vi "PI Open Interface of one system.vi"(0 "System number":i32=1 min=1 step=1, 2 "Interface clear":string="XXX\n", 3 "Interface configuration":T10={"RS232 Portnumber"=0, "Timeout"=5000, "RS232 Baud rate"=57600, "Interface"=0, "GPIB Bus"=0, "GPIB Address"=4, "GPIB Mode"=0} {"Interface" items=["RS232", "GPIB", "DLL", "TCP-IP", "USB", "Analog"]; "RS232 Portnumber" items=["COM1", "COM2", "COM3", "COM4", "COM5", "COM6", "COM7", "COM8", "COM9", "COM10", "COM11", "COM12", "COM13", "COM14", "COM15", "COM16", "COM17", "COM18", "COM19", "COM20", "COM21", "COM22", "COM23", "COM24", "COM25", "COM26", "COM27", "COM28", "COM29", "COM30"]}, 4 "String to Send":string="*idn?", 5 "error in":errorcluster, 6 "DLL Interface\nConfiguration":T8={"DLL for Device"=0, "DLL Interface"=2, "Parameter"="1"} {"DLL Interface" items=["RS232", "GPIB", "Board", "TCP-IP", "USB", "RS232_DC", "USB_DC", "TCPIP_DC"]; "DLL for Device" items=["C-843", "C-844", "E-710", "C-843.PM", "C-865", "E-761", "Mercury", "E-755", "E-753", "C-866", "E-712", "E-725", "E-861", "C-867", "E-517", "E-816", "E-709", "PI_GCS2_DLL", "HydraPollux"]}, 7 "Bit settings and parity":T4={"data bits"=8, "stop bits"=enum."1 bit", "parity"=enum."no parity"} {"data bits" min=5 max=8 step=1}, 8 "TCP/IP\nConfiguration":T3={"Host address/name"="localhost", "Port"=3000, "Board"=0}, 9 "Flow control":T5={"input XON/XOFF"=FALSE, "input HW Handshake"=FALSE, "input alt HW HShk"=FALSE, "output XON/XOFF"=FALSE, "output HW Handshake"=FALSE, "output alt HW HShk"=FALSE, "XOFF byte "=19, "XON byte"=17, "parity error byte"=0} {"parity error byte" format="%.0x"; "XON byte" format="%.0x"; "XOFF byte" format="%.0x"}, 10 "Termination character":T2, 11 "Syntax":T1, 12 "Register DC":bool) -> (14 "String read":string, 19 "error out":errorcluster)   [LabVIEW 2020]
doc: "Establishes communication with one connected system. This VI is called automatically by PI_GCS2_Configuration_Setup.vi and must be completed successfully before any other VI can use the interface. The interface and error status of the chosen system are cleared by this VI, which sends XXX (no command), *IDN? and ERR?. \n\nC-413: Interface = RS232, DLL, or TCP/IP (TCP/IP support available depending on controller version! If unsure whether your controller supports TCP/IP communication, please refer to the controller user manual). RS232: Input and output HW handshake must be TRUE. DLL: DLL for Device = PI_GCS2_DLL, DLL Interface = USB, Parameter = Serial no. of system to connect to. Syntax: GCS 2.0; Term char = LF.\n\nC-702: Interface = RS232 or TCP/IP, RS232: Input and output HW handshake must be TRUE, Syntax: GCS 1.0; Term char = LF.\n\nC-843: Interface = DLL, DLL for Device = C-843, DLL Interface = Board, Parameter = Board number (1 for first C-843 board), Syntax: GCS 1.0; Term char = LF.\n\nC-843.PM: Interface = DLL, DLL for Device = C-843.PM, DLL Interface = Board, Parameter = Board number (1 for first C-843 board) , Syntax: GCS 1.0; Term char = LF.\n\nC-844: Interface = DLL, DLL for Device = C-844, DLL Interface = RS232 or GPIB, Parameter = empty string, RS232 baud rate = 9600\n\nC-865: Interface = DLL, DLL for Device = C-865, DLL Interface = RS232, Parameter = empty string, RS232 baud rate = set as appropriate, Syntax: GCS 1.0; Term char = LF.\n\nC-866: Interface = DLL, DLL for Device = C-866, DLL Interface = RS232 or USB, RS232: Parameter = empty string, RS232 baud rate = set as appropriate, USB: Parameter = Serial no. of system to connect to, \nSyntax: GCS 1.0; Term char = LF.\n\nC-867: Single Device: Interface = RS232, TCP/IP or DLL, RS232: Input and output HW handshake must be FALSE. DLL (USB): DLL for Device = C-867, DLL Interface = USB, Parameter = Serial no. of system to connect to.\nDaisyChain: Interface = DLL, DLL for Device = C-867, DLL Interface = RS232_DC, Parameter = Number of device in chain, Register DC: FALSE. Syntax: GCS 2.0; Term char = LF.\n\nC-877: Interface = RS232 or DLL, RS232: Input and output HW handshake must be FALSE. DLL (USB): DLL for Device = PI_GCS2_DLL, DLL Interface = USB, Parameter = Serial no. of system to connect to. Syntax: GCS 2.0; Term char = LF.\n\nC-880: Interface = RS232 or GPIB, RS232: Input and output HW handshake must be TRUE, Syntax: GCS 1.0; Term char = LF.\n\nC-848: Interface = RS232 or GPIB, RS232: Input and output HW handshake must be TRUE, Syntax: GCS 1.0; Term char = LF.\n\nC-880K005: Interface = RS232, Input and output HW handshake must be FALSE, Syntax: GCS 1.0; Term char = LF.\n\nC-884: Interface = RS232, TCP/IP or DLL, RS232: Input and output HW handshake must be TRUE. DLL (USB): DLL for Device = PI_GCS2_DLL, DLL Interface = USB, Parameter = Serial no. of system to connect to. Syntax: GCS 2.0; Term char = LF.\n\nC-885: Interface = TCP/IP or DLL. DLL (USB): DLL for Device = PI_GCS2_DLL, DLL Interface = USB, Parameter = Serial no. of system to connect to. Syntax: GCS 2.0; Term char = LF.DaisyChain: Interface = DLL, DLL for Device = PI_GCS2_DLL, DLL Interface = TCPIP_DC or USB_DC, Parameter = Number of device in chain, Register DC: FALSE. Syntax: GCS 2.0; Term char = LF.\n\nC-886: Interface = TCP/IP or DLL. DLL (USB): DLL for Device = PI_GCS2_DLL, DLL Interface = USB, Parameter = Serial no. of system to connect to. Syntax: GCS 2.0; Term char = LF.\n\nC-891: Interface = RS232, TCP/IP or DLL. TCP/IP support available depending on controller version! If unsure whether your controller supports TCP/IP communication, please refer to your user manual.RS232: Input and output HW handshake must be FALSE. DLL: DLL for Device = C-891, DLL Interface = USB, Parameter = Serial no. of system to connect to. Syntax: GCS 2.0; Term char = LF.\n\nE-135: Interface = RS232, DLL, or TCP/IP. RS232: Input and output HW handshake must be TRUE. DLL: DLL for Device = PI_GCS2_DLL, DLL Interface = USB, Parameter = Serial no. of system to connect to. Syntax: GCS 2.0; Term char = LF.\n\nE-516: Interface = RS232 or GPIB, RS232: Input and output HW handshake must be TRUE, Syntax: GCS 1.0; Term char = LF.\n\nE-517: Interface = RS232, GPIB, TCP/IP or DLL, RS232: Input and output HW handshake must be TRUE, DLL (USB): DLL for Device = E-517, DLL Interface = USB, Parameter = Serial no. of system to connect to. Syntax: GCS 2.0; Term char = LF.\n\nE-518: Interface = RS232, TCP/IP or DLL, RS232: Input and output HW handshake must be TRUE, DLL (USB): DLL for Device = PI_GCS2_DLL, DLL Interface = SB, Parameter = Serial no. of system to connect to. Syntax: GCS 2.0; Term char = LF.\n\nE-709: Interface = RS232 or USB, RS232: Input and output HW handshake must be TRUE, DLL: DLL for Device = E-709, DLL Interface = USB, Parameter = Serial no. of system to connect to. \nSyntax: GCS 2.0; Term char = LF.\n\nE-710: Interface = DLL, DLL for Device = E-710, DLL Interface = RS232 or GPIB, Parameter = empty string, Syntax: GCS 1.0; Term char = LF.\n\nE-712: Interface = RS232, TCP/IP or DLL, RS232: Input and output HW handshake must be TRUE. DLL: DLL for Device = E-712, DLL Interface = USB, Parameter = Serial no. of system to connect to. Syntax: GCS 2.0; Term char = LF.\n\nE-725: Interface = RS232, TCP/IP or DLL, RS232: Input and output HW handshake must be TRUE. DLL: DLL for Device = E-725, DLL Interface = USB, Parameter = Serial no. of system to connect to. Syntax: GCS 2.0; Term char = LF.\n\nE-727: Interface = RS232, TCP/IP or DLL, RS232: Input and output HW handshake must be TRUE. DLL: DLL for Device = PI_GCS2_DLL, DLL Interface = USB, arameter = Serial no. of system to connect to. Syntax: GCS 2.0; Term char = LF.\n\nE-753: Interface = RS232 or TCP/IP, RS232: Input and output HW handshake must be TRUE, Syntax: GCS 2.0; Term char = LF.\n\nE-754: Interface = RS232, TCP/IP or DLL, RS232: Input and output HW handshake must be TRUE. DLL: DLL for Device = E-754, DLL Interface = USB, Parameter = Serial no. of system to connect to. Syntax: GCS 2.0; Term char = LF.\n\nE-755: Single Device: Interface = RS232, Input and output HW handshake must be TRUE.\nDaisyChain: Interface = DLL, DLL for Device = E-755, DLL Interface = RS232_DC, Parameter = Number of device in chain (first device: 1), Register DC: FALSE.\nSyntax: GCS 2.0; Term char = LF.\n\nE-761: Interface = DLL, DLL for Device = E-761, DLL Interface = Board, Parameter = Board number (1 for first E-761 board), Syntax: GCS 1.0; Term char = LF.\n\nE-816: Interface = RS232 or DLL, RS232: Input and output HW handshake must be TRUE. DLL (USB): DLL for Device = E-816, DLL Interface = USB, Parameter = Serial no. of system to connect to. Syntax: GCS 1.0; Term char = LF. \n\nE-861: Single Device: Interface = RS232 or DLL, RS232: Input and output HW handshake must be FALSE. DLL (USB): DLL for Device = E-861, DLL Interface = USB, Parameter = Serial no. of system to connect to.\nDaisyChain: Interface = DLL, DLL for Device = E-861, DLL Interface = RS232_DC or USB_DC, Parameter = Number of device in chain, Register DC: FALSE. Syntax: GCS 2.0; Term char = LF.\n\nE-870: Interface = DLL, DLL (USB): DLL for Device = PI_GCS2_DLL, DLL Interface = USB, Parameter = Serial no. of system to connect to. Syntax: GCS 2.0; Term char = LF. \n\nE-871: Single Device: Interface = RS232 or DLL, RS232: Input and output HW handshake must be FALSE. DLL (USB): DLL for Device = PI_GCS2_DLL, DLL Interface = USB, Parameter = Serial no. of system to connect to.\nDaisyChain: Interface = DLL, DLL for Device = PI_GCS2_DLL, DLL Interface = RS232_DC or USB_DC, Parameter = Number of device in chain, Register DC: FALSE. Syntax: GCS 2.0; Term char = LF.\n\nE-872: Interface = RS232, TCP/IP or DLL, RS232: Input and output HW handshake must be FALSE. DLL (USB): DLL for Device = PI_GCS2_DLL, DLL Interface = USB, Parameter = Serial no. of system to connect to. Syntax: GCS 2.0; Term char = LF.\n\nE-873: Interface = RS232, TCP/IP or DLL, RS232: Input and output HW handshake must be FALSE. DLL (USB): DLL for Device = PI_GCS2_DLL, DLL Interface = USB, Parameter = Serial no. of system to connect to. Syntax: GCS 2.0; Term char = LF.\n\nE-874: Interface = RS232, TCP/IP or DLL, RS232: Input and output HW handshake must be FALSE. DLL (USB): DLL for Device = PI_GCS2_DLL, DLL Interface = USB, Parameter = Serial no. of system to connect to. Syntax: GCS 2.0; Term char = LF.\n\nF-206: F-206 (GCS 1.0): Interface = RS232, GPIB or TCP/IP, The error status will not be cleared by this VI. The first ERR? query will report a hidden error with error code 1, which will be cleared during system initialization (INI). RS232: Input and output handshake settings must be FALSE, Syntax: GCS 1.0; Term char = LF.\n\nC-887 + H-206 (GCS 2.0): Interface = RS232 or TCP/IP, RS232: Input and output handshake settings must be FALSE, Syntax: GCS 2.0; Term char = LF.\n\nHydra: Interface = DLL, DLL (TCP/IP and RS-232): DLL for Device = PI_HydraPollux_GCS2_DLL, DLL Interface = RS232 or TCP/IP, Syntax: GCS 2.0; Term char = LF. \n\nM-8X0: M-810/11/24/40/50 (GCS 1.0): Interface = RS232, GPIB or TCP/IP, RS232: Input and output handshake settings must be FALSE, Syntax: GCS 1.0; Term char = LF.\n\nC-887 + H-810/11/24/40/50 (GCS 2.0): Interface = RS232 or TCP/IP, RS232: Input and output handshake settings must be FALSE, Syntax: GCS 2.0; Term char = LF.\n\nMercury: Interface = DLL, DLL for Device = Mercury, DLL Interface = RS232 (even if using USB), Parameter = empty string, RS232 baud rate = same as controller hardware setting (even if using USB), Syntax: GCS 1.0; Term char = LF.\n\nMercury_GCS: Single Device: Interface = RS232 or DLL, RS232: Input and output HW handshake must be FALSE. DLL (USB): DLL for Device = PI_GCS2_DLL, DLL Interface = USB, Parameter = Serial no. of system to connect to.\nDaisyChain: Interface = DLL, DLL for Device = PI_GCS2_DLL, DLL Interface = RS232_DC or USB_DC, Parameter = Number of device in chain, Register DC: FALSE. Syntax: GCS 2.0; Term char = LF.\n\nPollux: Interface = DLL, DLL (RS-232): DLL for Device = PI_HydraPollux_GCS2_DLL, DLL Interface = RS232, Baudrate must be 19200. Syntax: GCS 2.0; Term char = LF."
uses:
  Available interfaces.ctl
  Available DLLs.ctl
  Available DLL interfaces.ctl
  Termination character.ctl
  Syntax.ctl
  Global1.vi
  <vilib>/Instr/_visa.llb/VISA Configure Serial Port (Instr).vi
panel:
  out "DLL device ID":i32 caption="error code"
  # "Establishes communication with one connected system. This VI is called automatically by \"XXXX_\nConfiguration_Setup.vi\" (with XXXX being the PI product number of your system) and must be \ncompleted successfully before any other VI can use the interface. The interface and error status \nof the chosen system are cleared by this VI, which sends XXX (no command), *IDN? and ERR?. \nOther system entries are not touched."
  # "Other parameters:"
  # "TCP/IP:"
  # "DLL:"
  # "General:"
  # "RS232:"
  # "GPIB:"
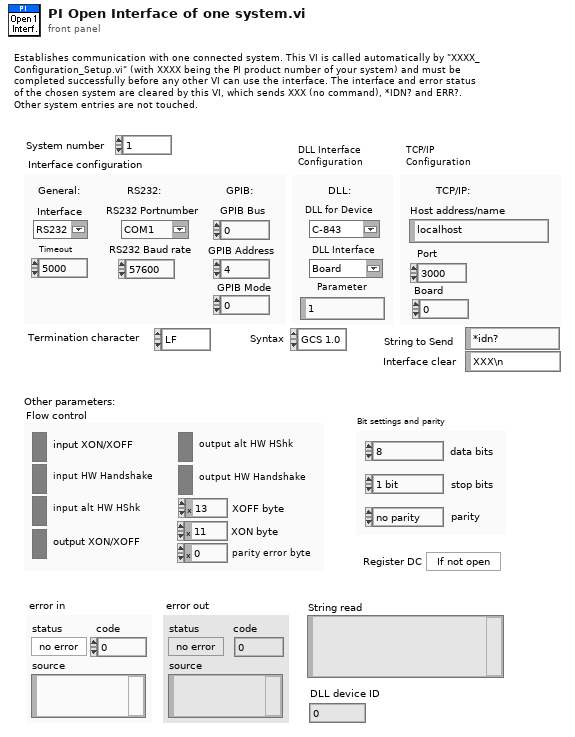
[diagram p1: front panel]
types:
  T1 = typedef "Syntax.ctl" = enum16{"GCS 1.0", "GCS 2.0", "GCS 3.0"}
  T2 = typedef "Termination character.ctl" = enum16{"LF", "CR", "LFCR", "CRLF"}
  T3 = cluster{"Host address/name":string, "Port":i32, "Board":i32}
  T4 = cluster{"data bits":u16, "stop bits":enum16{"1 bit", "1.5 bits", "2 bits"}, "parity":enum16{"no parity", "odd parity", "even parity", "mark parity", "space parity"}}
  T5 = cluster{"input XON/XOFF":bool, "input HW Handshake":bool, "input alt HW HShk":bool, "output XON/XOFF":bool, "output HW Handshake":bool, "output alt HW HShk":bool, "XOFF byte ":u8, "XON byte":u8, "parity error byte":u16}
  T6 = typedef "Available DLLs.ctl" = u16
  T7 = typedef "Available DLL interfaces.ctl" = u16
  T8 = cluster{"DLL for Device":T6, "DLL Interface":T7, "Parameter":string}
  T9 = typedef "Available interfaces.ctl" = u16
  T10 = cluster{"RS232 Portnumber":i32, "Timeout":i32, "RS232 Baud rate":u32, "Interface":T9, "GPIB Bus":i32, "GPIB Address":i32, "GPIB Mode":i32}
  T11 = enum16{"C844_IsDLLAvailable", "C844_ConnectRS232", "C844_ConnectNIgpib", "C844_IsConnected", "C844_CloseConnection", "C844_GcsCommandset", "C844_GetError", "C844_GcsGetAnswerSize", "C844_GcsGetAnswer", "C843_IsDLLAvailable", "C843_Connect", "C843_IsConnected", "C843_CloseConnection", "C843_GcsCommandset", "C843_GetError", "C843_GcsGetAnswerSize", "C843_GcsGetAnswer", "E710_IsDLLAvailable", "E710_ConnectRS232", "E710_ConnectNIgpib", "E710_IsConnected", "E710_CloseConnection", "E710_GcsCommandset", "E710_GetError", "E710_GcsGetAnswerSize", "E710_GcsGetAnswer", "C843_PM_IsDLLAvailable", "C843_PM_Connect", "C843_PM_IsConnected", "C843_PM_CloseConnection", "C843_PM_GcsCommandset", "C843_PM_GetError", "C843_PM_GcsGetAnswerSize", "C843_PM_GcsGetAnswer", "C843_PM_GetCurrentBoardID", "C843_GetCurrentBoardID", "C865_IsDLLAvailable", "C865_ConnectRS232", "C865_IsConnected", "C865_CloseConnection", "C865_GcsCommandset", "C865_GetError", "C865_GcsGetAnswerSize", "C865_GcsGetAnswer", "C865_GetCurrentInterfaceID", "E761_ConnectPciBoard", "DefineSystem", "CloseConnection", "IsConnected", "ConnectRS232", "ConnectNIgpib", "ConnectPciBoard", "ConnectTCPIP", "GetError", "GcsCommandset", "GCSGetAnswerSize", "GcsGetAnswer"}
  T12 = enum16{"C844_IsDLLAvailable", "C844_ConnectRS232", "C844_ConnectNIgpib", "C844_IsConnected", "C844_CloseConnection", "C844_GcsCommandset", "C844_GetError", "C844_GcsGetAnswerSize", "C844_GcsGetAnswer", "C843_IsDLLAvailable", "C843_Connect", "C843_IsConnected", "C843_CloseConnection", "C843_GcsCommandset", "C843_GetError", "C843_GcsGetAnswerSize", "C843_GcsGetAnswer", "E710_IsDLLAvailable", "E710_ConnectRS232", "E710_ConnectNIgpib", "E710_IsConnected", "E710_CloseConnection", "E710_GcsCommandset", "E710_GetError", "E710_GcsGetAnswerSize", "E710_GcsGetAnswer", "C843_PM_IsDLLAvailable", "C843_PM_Connect", "C843_PM_IsConnected", "C843_PM_CloseConnection", "C843_PM_GcsCommandset", "C843_PM_GetError", "C843_PM_GcsGetAnswerSize", "C843_PM_GcsGetAnswer", "C843_PM_GetCurrentBoardID", "C843_GetCurrentBoardID", "C865_IsDLLAvailable", "C865_ConnectRS232", "C865_IsConnected", "C865_CloseConnection", "C865_GcsCommandset", "C865_GetError", "C865_GcsGetAnswerSize", "C865_GcsGetAnswer", "C865_GetCurrentInterfaceID", "E761_ConnectPciBoard", "DefineSystem", "CloseConnection", "IsConnected", "ConnectRS232", "ConnectNIgpib", "ConnectPciBoard", "ConnectTCPIP", "GetError", "GcsCommandset", "GCSGetAnswerSize", "GcsGetAnswer", "CloseDaisyChain", "OpenRS232DaisyChain", "ConnectDaisyChainDevice", "ConnectUSB", "ListUSB"}
  T13 = enum16{"C844_IsDLLAvailable", "C844_ConnectRS232", "C844_ConnectNIgpib", "C844_IsConnected", "C844_CloseConnection", "C844_GcsCommandset", "C844_GetError", "C844_GcsGetAnswerSize", "C844_GcsGetAnswer", "C843_IsDLLAvailable", "C843_Connect", "C843_IsConnected", "C843_CloseConnection", "C843_GcsCommandset", "C843_GetError", "C843_GcsGetAnswerSize", "C843_GcsGetAnswer", "E710_IsDLLAvailable", "E710_ConnectRS232", "E710_ConnectNIgpib", "E710_IsConnected", "E710_CloseConnection", "E710_GcsCommandset", "E710_GetError", "E710_GcsGetAnswerSize", "E710_GcsGetAnswer", "C843_PM_IsDLLAvailable", "C843_PM_Connect", "C843_PM_IsConnected", "C843_PM_CloseConnection", "C843_PM_GcsCommandset", "C843_PM_GetError", "C843_PM_GcsGetAnswerSize", "C843_PM_GcsGetAnswer", "C843_PM_GetCurrentBoardID", "C843_GetCurrentBoardID", "C865_IsDLLAvailable", "C865_ConnectRS232", "C865_IsConnected", "C865_CloseConnection", "C865_GcsCommandset", "C865_GetError", "C865_GcsGetAnswerSize", "C865_GcsGetAnswer", "C865_GetCurrentInterfaceID", "E761_ConnectPciBoard", "DefineSystem", "CloseConnection", "IsConnected", "ConnectRS232", "ConnectNIgpib", "ConnectPciBoard", "ConnectTCPIP", "GetError", "GcsCommandset", "GCSGetAnswerSize", "GcsGetAnswer", "CloseDaisyChain", "OpenRS232DaisyChain", "ConnectDaisyChainDevice"}
  T14 = enum16{"C844_IsDLLAvailable", "C844_ConnectRS232", "C844_ConnectNIgpib", "C844_IsConnected", "C844_CloseConnection", "C844_GcsCommandset", "C844_GetError", "C844_GcsGetAnswerSize", "C844_GcsGetAnswer", "C843_IsDLLAvailable", "C843_Connect", "C843_IsConnected", "C843_CloseConnection", "C843_GcsCommandset", "C843_GetError", "C843_GcsGetAnswerSize", "C843_GcsGetAnswer", "E710_IsDLLAvailable", "E710_ConnectRS232", "E710_ConnectNIgpib", "E710_IsConnected", "E710_CloseConnection", "E710_GcsCommandset", "E710_GetError", "E710_GcsGetAnswerSize", "E710_GcsGetAnswer", "C843_PM_IsDLLAvailable", "C843_PM_Connect", "C843_PM_IsConnected", "C843_PM_CloseConnection", "C843_PM_GcsCommandset", "C843_PM_GetError", "C843_PM_GcsGetAnswerSize", "C843_PM_GcsGetAnswer", "C843_PM_GetCurrentBoardID", "C843_GetCurrentBoardID", "C865_IsDLLAvailable", "C865_ConnectRS232", "C865_IsConnected", "C865_CloseConnection", "C865_GcsCommandset", "C865_GetError", "C865_GcsGetAnswerSize", "C865_GcsGetAnswer", "C865_GetCurrentInterfaceID", "E761_ConnectPciBoard", "DefineSystem", "CloseConnection", "IsConnected", "ConnectRS232", "ConnectNIgpib", "ConnectPciBoard", "ConnectTCPIP", "GetError", "GcsCommandset", "GCSGetAnswerSize", "GcsGetAnswer", "CloseDaisyChain", "OpenRS232DaisyChain", "ConnectDaisyChainDevice", "ConnectUSB", "ListUSB", "OpenUSBDaisyChain"}
  T15 = enum16{"C844_IsDLLAvailable", "C844_ConnectRS232", "C844_ConnectNIgpib", "C844_IsConnected", "C844_CloseConnection", "C844_GcsCommandset", "C844_GetError", "C844_GcsGetAnswerSize", "C844_GcsGetAnswer", "C843_IsDLLAvailable", "C843_Connect", "C843_IsConnected", "C843_CloseConnection", "C843_GcsCommandset", "C843_GetError", "C843_GcsGetAnswerSize", "C843_GcsGetAnswer", "E710_IsDLLAvailable", "E710_ConnectRS232", "E710_ConnectNIgpib", "E710_IsConnected", "E710_CloseConnection", "E710_GcsCommandset", "E710_GetError", "E710_GcsGetAnswerSize", "E710_GcsGetAnswer", "C843_PM_IsDLLAvailable", "C843_PM_Connect", "C843_PM_IsConnected", "C843_PM_CloseConnection", "C843_PM_GcsCommandset", "C843_PM_GetError", "C843_PM_GcsGetAnswerSize", "C843_PM_GcsGetAnswer", "C843_PM_GetCurrentBoardID", "C843_GetCurrentBoardID", "C865_IsDLLAvailable", "C865_ConnectRS232", "C865_IsConnected", "C865_CloseConnection", "C865_GcsCommandset", "C865_GetError", "C865_GcsGetAnswerSize", "C865_GcsGetAnswer", "C865_GetCurrentInterfaceID", "E761_ConnectPciBoard", "DefineSystem", "CloseConnection", "IsConnected", "ConnectRS232", "ConnectNIgpib", "ConnectPciBoard", "ConnectTCPIP", "GetError", "GcsCommandset", "GCSGetAnswerSize", "GcsGetAnswer", "CloseDaisyChain", "OpenRS232DaisyChain", "ConnectDaisyChainDevice", "ConnectUSB", "ListUSB", "OpenUSBDaisyChain", "OpenTCPIPDaisyChain"}
  T16 = enum16{"C844_IsDLLAvailable", "C844_ConnectRS232", "C844_ConnectNIgpib", "C844_IsConnected", "C844_CloseConnection", "C844_GcsCommandset", "C844_GetError", "C844_GcsGetAnswerSize", "C844_GcsGetAnswer", "C843_IsDLLAvailable", "C843_Connect", "C843_IsConnected", "C843_CloseConnection", "C843_GcsCommandset", "C843_GetError", "C843_GcsGetAnswerSize", "C843_GcsGetAnswer"}
  T17 = enum16{"C844_IsDLLAvailable", "C844_ConnectRS232", "C844_ConnectNIgpib", "C844_IsConnected", "C844_CloseConnection", "C844_GcsCommandset", "C844_GetError", "C844_GcsGetAnswerSize", "C844_GcsGetAnswer"}
  T18 = enum16{"C844_IsDLLAvailable", "C844_ConnectRS232", "C844_ConnectNIgpib", "C844_IsConnected", "C844_CloseConnection", "C844_GcsCommandset", "C844_GetError", "C844_GcsGetAnswerSize", "C844_GcsGetAnswer", "C843_IsDLLAvailable", "C843_Connect", "C843_IsConnected", "C843_CloseConnection", "C843_GcsCommandset", "C843_GetError", "C843_GcsGetAnswerSize", "C843_GcsGetAnswer", "E710_IsDLLAvailable", "E710_ConnectRS232", "E710_ConnectNIgpib", "E710_IsConnected", "E710_CloseConnection", "E710_GcsCommandset", "E710_GetError", "E710_GcsGetAnswerSize", "E710_GcsGetAnswer", "C843_PM_IsDLLAvailable", "C843_PM_Connect", "C843_PM_IsConnected", "C843_PM_CloseConnection", "C843_PM_GcsCommandset", "C843_PM_GetError", "C843_PM_GcsGetAnswerSize", "C843_PM_GcsGetAnswer", "C843_PM_GetCurrentBoardID", "C843_GetCurrentBoardID", "C865_IsDLLAvailable", "C865_ConnectRS232", "C865_IsConnected", "C865_CloseConnection", "C865_GcsCommandset", "C865_GetError", "C865_GcsGetAnswerSize", "C865_GcsGetAnswer", "C865_GetCurrentInterfaceID"}
  T19 = enum16{"C844_IsDLLAvailable", "C844_ConnectRS232", "C844_ConnectNIgpib", "C844_IsConnected", "C844_CloseConnection", "C844_GcsCommandset", "C844_GetError", "C844_GcsGetAnswerSize", "C844_GcsGetAnswer", "C843_IsDLLAvailable", "C843_Connect", "C843_IsConnected", "C843_CloseConnection", "C843_GcsCommandset", "C843_GetError", "C843_GcsGetAnswerSize", "C843_GcsGetAnswer", "E710_IsDLLAvailable", "E710_ConnectRS232", "E710_ConnectNIgpib", "E710_IsConnected", "E710_CloseConnection", "E710_GcsCommandset", "E710_GetError", "E710_GcsGetAnswerSize", "E710_GcsGetAnswer"}
  T20 = enum16{"C844_IsDLLAvailable", "C844_ConnectRS232", "C844_ConnectNIgpib", "C844_IsConnected", "C844_CloseConnection", "C844_GcsCommandset", "C844_GetError", "C844_GcsGetAnswerSize", "C844_GcsGetAnswer", "C843_IsDLLAvailable", "C843_Connect", "C843_IsConnected", "C843_CloseConnection", "C843_GcsCommandset", "C843_GetError", "C843_GcsGetAnswerSize", "C843_GcsGetAnswer", "E710_IsDLLAvailable", "E710_ConnectRS232", "E710_ConnectNIgpib", "E710_IsConnected", "E710_CloseConnection", "E710_GcsCommandset", "E710_GetError", "E710_GcsGetAnswerSize", "E710_GcsGetAnswer", "C843_PM_IsDLLAvailable", "C843_PM_Connect", "C843_PM_IsConnected", "C843_PM_CloseConnection", "C843_PM_GcsCommandset", "C843_PM_GetError", "C843_PM_GcsGetAnswerSize", "C843_PM_GcsGetAnswer"}
  T21 = cluster{"DLL for Device":T6, "DLL Interface":T7, "Parameter":string}[]
  T22 = cluster{"Host address/name":string, "Port":i32, "Board":i32}[]
  T23 = cluster{"RS232 Portnumber":i32, "Timeout":i32, "RS232 Baud rate":u32, "Interface":T9, "GPIB Bus":i32, "GPIB Address":i32, "GPIB Mode":i32}[]
  T24 = cluster{"data bits":u16, "stop bits":enum16{"1 bit", "1.5 bits", "2 bits"}, "parity":enum16{"no parity", "odd parity", "even parity", "mark parity", "space parity"}}[]
  T25 = cluster{"input XON/XOFF":bool, "input HW Handshake":bool, "input alt HW HShk":bool, "output XON/XOFF":bool, "output HW Handshake":bool, "output alt HW HShk":bool, "XOFF byte ":u8, "XON byte":u8, "parity error byte":u16}[]
  T26 = enum16{"no parity", "odd parity", "even parity", "mark parity", "space parity"}
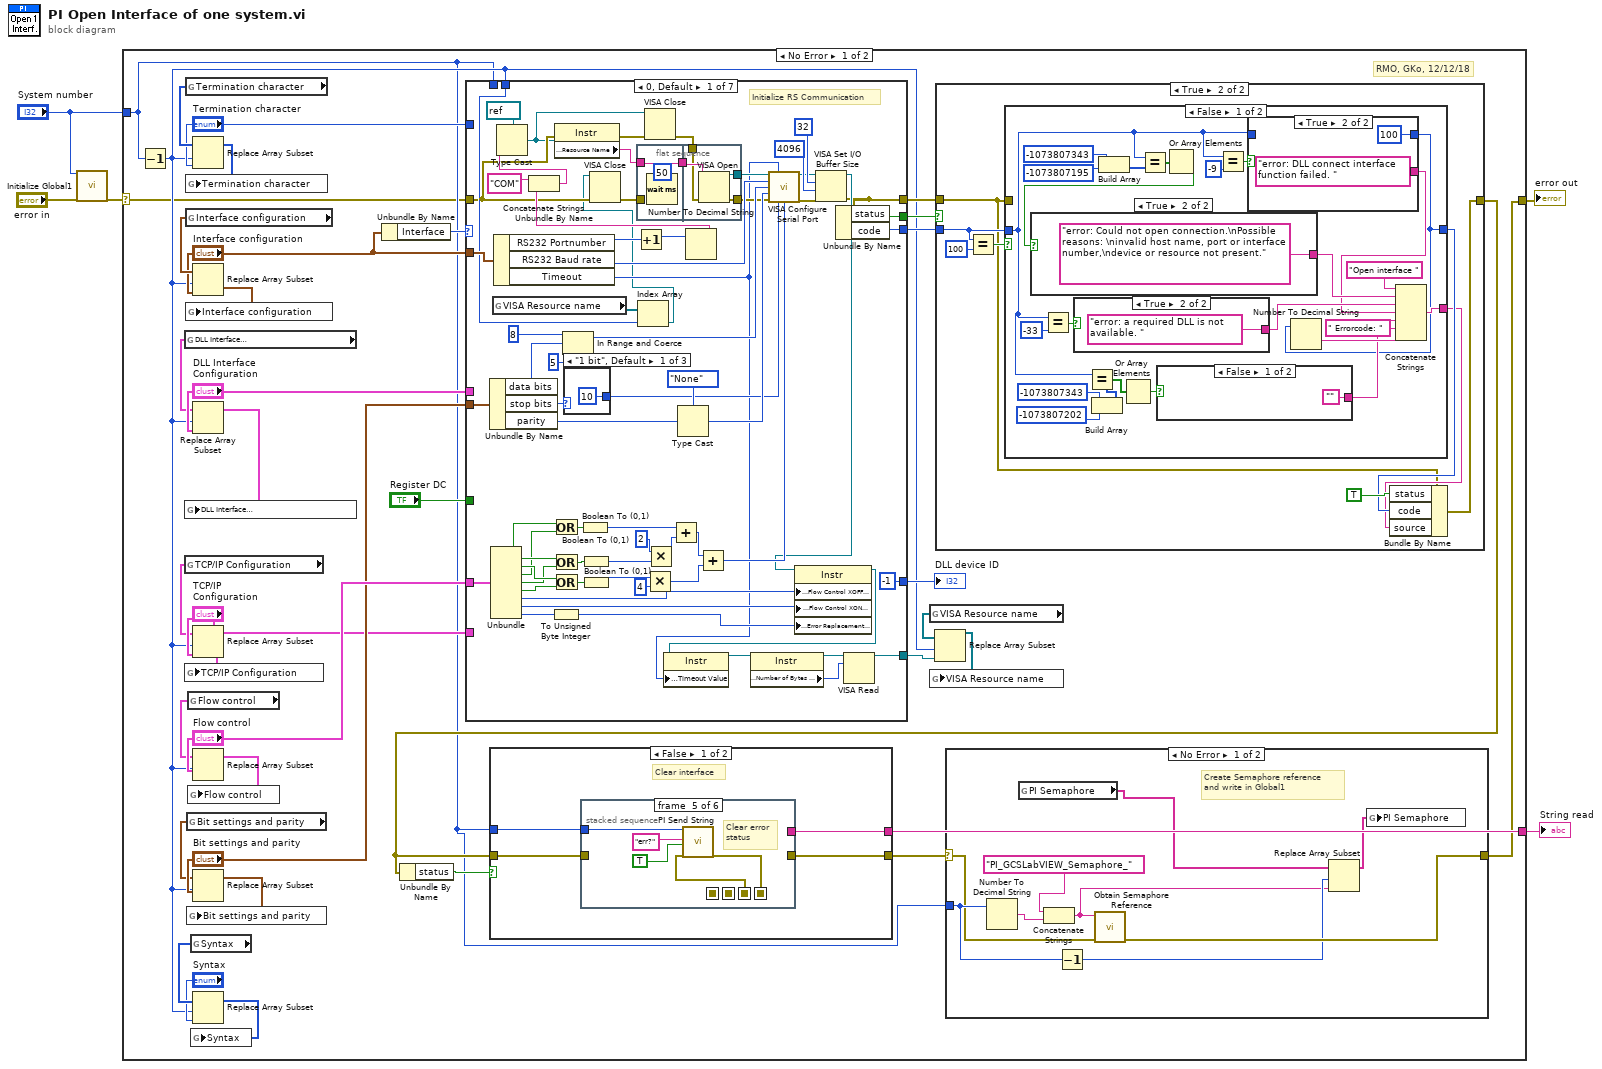
[diagram p0: block diagram]
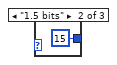
[diagram p3: hidden frame]
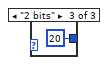
[diagram p4: hidden frame]
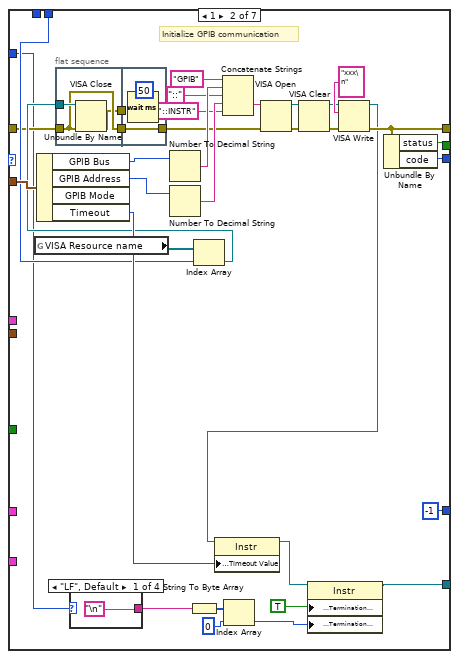
[diagram p5: hidden frame]
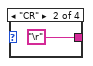
[diagram p6: hidden frame]
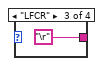
[diagram p7: hidden frame]
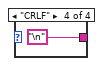
[diagram p8: hidden frame]
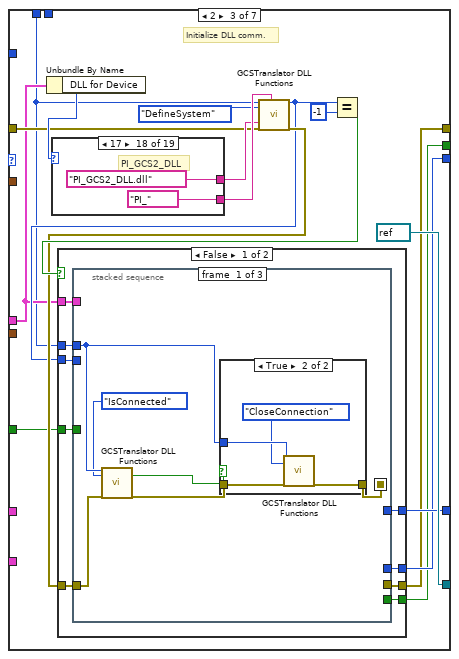
[diagram p9: hidden frame]
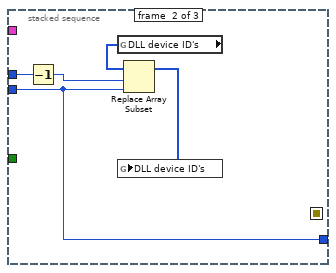
[diagram p11: hidden frame]
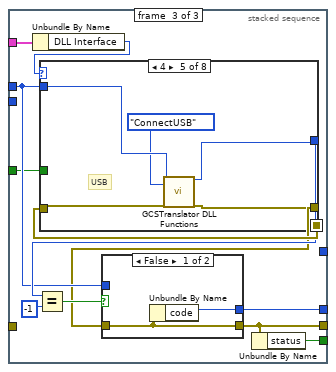
[diagram p12: hidden frame]
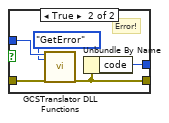
[diagram p13: hidden frame]
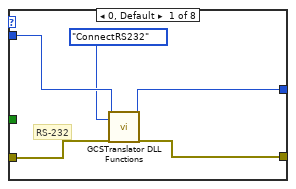
[diagram p14: hidden frame]
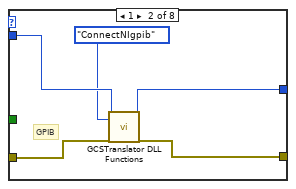
[diagram p15: hidden frame]
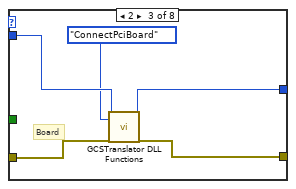
[diagram p16: hidden frame]
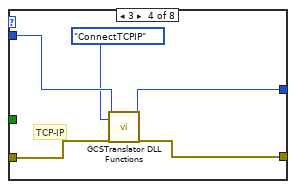
[diagram p17: hidden frame]
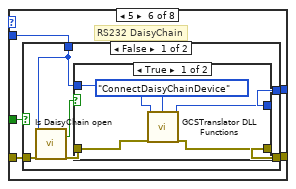
[diagram p18: hidden frame]
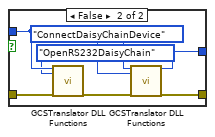
[diagram p19: hidden frame]
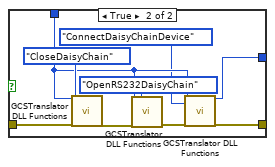
[diagram p20: hidden frame]
diagram:
  n1 = call "Initialize Global1.vi"("System no."="System number", "error in"="error in") -> ("error out"=w1:errorcluster)  [unwired: 17 out]
  n2 = case shown="No Error" w1 {
    selector: w1 -> [w6 w906]
    tunnel: [w8 w906] -> w4
    tunnel: [w29 "" ("String read")] -> w5
    tunnel: "System number" -> [w9 _]
    frame No Error {
      # "RMO, GKo, 12/12/18"
      n3 = Decrement(x=w9) -> (x-1=w11:i32)
      n4 = global read "Global1.vi" "DLL Interface\nConfiguration"() -> (w34:T21)
      n5 = global read "Global1.vi" "TCP/IP Configuration"() -> (w25:T22)
      n6 = global read "Global1.vi" "Termination character"() -> (w18:T2[])
      n7 = global read "Global1.vi" "Interface configuration"() -> (w42:T23)
      n8 = global read "Global1.vi" "Bit settings and parity"() -> (w30:T24)
      n9 = global read "Global1.vi" "Flow control"() -> (w32:T25)
      n10 = global read "Global1.vi" "Syntax"() -> (w15:T1[])
      n11 = Replace Array Subset(array=w18, new element="Termination character", index=w11) -> (w17:T2[])
      n12 = global write "Global1.vi" "Termination character"(w17) -> ()
      n13 = Replace Array Subset(array=w42, new element="Interface configuration", index=w11) -> (w41:T23)
      n14 = global write "Global1.vi" "Interface configuration"(w41) -> ()
      n15 = Replace Array Subset(array=w34, new element="DLL Interface\nConfiguration", index=w11) -> (w38:T21)
      n16 = global write "Global1.vi" "DLL Interface\nConfiguration"(w38) -> ()
      n17 = Replace Array Subset(array=w25, new element="TCP/IP\nConfiguration", index=w11) -> (w21:T22)
      n18 = global write "Global1.vi" "TCP/IP Configuration"(w21) -> ()
      n19 = Replace Array Subset(array=w32, new element="Flow control", index=w11) -> (w33:T25)
      n20 = global write "Global1.vi" "Flow control"(w33) -> ()
      n21 = Replace Array Subset(array=w30, new element="Bit settings and parity", index=w11) -> (w31:T24)
      n22 = global write "Global1.vi" "Bit settings and parity"(w31) -> ()
      n23 = Replace Array Subset(array=w15, new element="Syntax", index=w11) -> (w14:T1[])
      n24 = global write "Global1.vi" "Syntax"(w14) -> ()
      n25 = Unbundle By Name("Interface configuration") -> ("Interface"=w40:T9)
      n26 = case shown="0, Default" w40 {
        tunnel: [w121 w154 w183 w422 0 0 w468] -> w19
        tunnel: "Interface configuration" -> [w119 w165 _ w425 _ _ _]
        tunnel: "DLL Interface\nConfiguration" -> [_ _ w179 _ _ _ w467]
        tunnel: w9 -> [_ _ w176 _ _ _ w461]
        tunnel: [w57 w147 w182 w416 errorcluster {"status"=TRUE, "code"=100, "source"="PI Open Interface of one system.vi:\nUSB interface not supported"} ("error out") w460 w466] -> w28
        tunnel: "Flow control" -> [w87 _ _ _ _ _ _]
        tunnel: "Bit settings and parity" -> [w118 _ _ _ _ _ _]
        tunnel: w6 -> [w65 w139 w187 w404 _ w460 w464]
        tunnel: "TCP/IP\nConfiguration" -> [_ _ _ w434 _ _ _]
        tunnel: [w79 w151 refnum<visa-resource-name> refnum ("duplicate VISA resource name") w423 refnum<visa-resource-name> refnum ("duplicate VISA resource name") refnum<visa-resource-name> refnum ("duplicate VISA resource name") refnum<visa-resource-name> refnum ("duplicate VISA resource name")] -> w22
        tunnel: [-1 -1 w185 -1 0 ("error code") 0 ("error code") w463] -> w20
        tunnel: "Termination character" -> [_ w133 _ w414 _ _ _]
        tunnel: [w72 w141 w178 w406 FALSE ("status") FALSE ("status") w462] -> w12
        tunnel: w11 -> [w71 w140 _ w405 _ _ _]
        tunnel: "Register DC" -> [_ _ w175 _ _ _ _]
        frame 0, Default {
          # "Initialize RS Communication"
          n27 = Unbundle By Name(w118) -> ("data bits"=w111:u16, "stop bits"=w110:enum16{"1 bit", "1.5 bits", "2 bits"}, "parity"=w116:T26)
          n28 = Unbundle(w87) -> ("input XON/XOFF"=w89:bool, "input HW Handshake"=w92:bool, "input alt HW HShk"=w94:bool, "output XON/XOFF"=w90:bool, "output HW Handshake"=w93:bool, "output alt HW HShk"=w95:bool, "XOFF byte"=w106:u8, "XON byte"=w107:u8, "parity error byte"=w88:u16)
          n29 = global read "Global1.vi" "VISA Resource name"() -> (w73:refnum<visa-resource-name>[])
          n30 = Unbundle By Name(w119) -> ("RS232 Portnumber"=w75:i32, "RS232 Baud rate"=w120:u32, "Timeout"=w78:i32)
          n31 = To Unsigned Byte Integer(number=w88) -> (unsigned 8bit integer=w108:u8)
          n32 = Or(x=w89, y=w90) -> (x .or. y?=w91:bool)
          n33 = Or(x=w92, y=w93) -> (x .or. y?=w96:bool)
          n34 = Or(x=w94, y=w95) -> (x .or. y?=w97:bool)
          n35 = In Range and Coerce(upper limit=u16 8, x=w111, lower limit=u16 5) -> (coerced(x)=w112:u16)  [unwired: 1 out]
          n36 = case shown="\"1 bit\", Default" w110 {
            tunnel: [u16 10 u16 15 u16 20] -> w109
            frame "1 bit", Default {
            }
            frame "1.5 bits" {
            }
            frame "2 bits" {
            }
          }
          n37 = Boolean To (0,1)(Boolean=w91) -> (0, 1=w102:i16)
          n38 = Boolean To (0,1)(Boolean=w96) -> (0, 1=w99:i16)
          n39 = Boolean To (0,1)(Boolean=w97) -> (0, 1=w101:i16)
          n40 = Increment(x=w75) -> (x+1=w76:i32)
          n41 = flat-sequence {
            tunnel: w74 -> [_]
            tunnel: w67 -> [w123]
            tunnel: [w123] -> w63
            tunnel: [w127] -> w83
            tunnel: [w126] -> w82
            tunnel: w63 -> [w125]
            tunnel: w54 -> [w124]
            frame #0 {
              n42 = Wait (ms)(milliseconds to wait=u32 50) -> ()  [unwired: 1 out]
            }
            frame #1 {
              n43 = VISA Open(error in (no error)=w124, VISA resource name=w125) -> (VISA resource name=w127:refnum<visa-resource-name>, error out=w126:errorcluster)  [unwired: 3 out]
            }
          }
          n44 = Index Array(array=w73, index=w71) -> (element=w64:refnum<visa-resource-name>)
          n45 = VISA Close(VISA resource name=w64, error in (no error)=w65) -> (error out=w74:errorcluster)
          n46 = Multiply(x=w101, y=u16 4) -> (x*y=w104:u16)
          n47 = Multiply(x=u16 2 ("y"), y=w99) -> (x*y=w103:u16)
          n48 = Add(x=w102, y=w103) -> (x+y=w105:u16)
          n49 = Type Cast(type=enum16{"None", "Odd", "Even", "Mark", "Space"}."None" ("parity (0:none)"), x=w116) -> (*(type *) &x=w115:enum16{"None", "Odd", "Even", "Mark", "Space"})
          n50 = Number To Decimal String(number=w76) -> (decimal integer string=w69:string)  [unwired: 1 out]
          n51 = Concatenate Strings("COM" ("string"), w69) -> (w66:string)
          n52 = Type Cast(type=refnum<visa-resource-name> refnum, x=w66) -> (*(type *) &x=w56:refnum<visa-resource-name>)
          n53 = property class="Instr"(reference=w56, error in=w65) -> (error out=w55:errorcluster, "General Settings:Resource Name"=w67:string)  [unwired: 1 out]
          n54 = VISA Close(VISA resource name=w56, error in (no error)=w55) -> (error out=w54:errorcluster)
          n55 = Add(x=w105, y=w104) -> (x+y=w86:u16)
          n56 = call-poly "VISA Configure Serial Port"("VISA resource name"=w83, "timeout (10sec)"=w78, "baud rate (9600)"=w120, "data bits (8)"=w112, "parity (0:none)"=w115, "error in (no error)"=w82, "stop bits (10: 1 bit)"=w109, "flow control (0:none)"=w86) -> ("VISA resource name out"=w60:refnum<visa-resource-name>, "error out"=w58:errorcluster)  [unwired: 6 out]
          n57 = VISA Set I/O Buffer Size(VISA resource name=w60, mask (16)=u16 32, size (4096)=u32 4096, error in (no error)=w58) -> (VISA resource name out=w59:refnum<visa-resource-name>, error out=w57:errorcluster)
          n58 = property class="Instr"(reference=w59, "Serial Settings:Flow Control XOFF Character"=w106, "Serial Settings:Flow Control XON Character"=w107, "Serial Settings:Error Replacement Character"=w108) -> (reference out=w81:refnum<visa-resource-name>)  [unwired: 1 in, 1 out]
          n59 = property class="Instr"(reference=w81, "General Settings:Timeout Value"=w78) -> (reference out=w80:refnum<visa-resource-name>)  [unwired: 1 in, 1 out]
          n60 = property class="Instr"(reference=w80) -> (reference out=w85:refnum<visa-resource-name>, "Serial Settings:Number of Bytes at Serial Port"=w84:u32)  [unwired: 1 in, 1 out]
          n61 = Unbundle By Name(w57) -> ("status"=w72:bool, "code"=w121:i32)
          n62 = VISA Read(VISA resource name=w85, byte count=w84) -> (VISA resource name out=w79:refnum<visa-resource-name>)  [unwired: 1 in, 3 out]
        }
        frame 1 {
          # "Initialize GPIB communication"
          n63 = global read "Global1.vi" "VISA Resource name"() -> (w144:refnum<visa-resource-name>[])
          n64 = Unbundle By Name(w165) -> ("GPIB Bus"=w164:i32, "GPIB Address"=w160:i32, "Timeout"=w153:i32)  [unwired: 1 out]
          n65 = flat-sequence {
            tunnel: w143 -> [w168]
            tunnel: w139 -> [w167]
            tunnel: [w167] -> w132
            tunnel: [w166] -> w131
            tunnel: [w170] -> w142
            tunnel: w132 -> [w170]
            tunnel: w131 -> [_]
            frame #0 {
              n66 = VISA Close(VISA resource name=w168, error in (no error)=w167) -> (error out=w166:errorcluster)
            }
            frame #1 {
              n67 = Wait (ms)(milliseconds to wait=u32 50) -> ()  [unwired: 1 out]
            }
          }
          n68 = case shown="\"LF\", Default" w133 {
            tunnel: ["\n" "\r" "\r" "\n"] -> w137
            frame "LF", Default {
            }
            frame "CR" {
            }
            frame "LFCR" {
            }
            frame "CRLF" {
            }
          }
          n69 = Number To Decimal String(number=w164) -> (decimal integer string=w162:string)  [unwired: 1 out]
          n70 = Number To Decimal String(number=w160) -> (decimal integer string=w159:string)  [unwired: 1 out]
          n71 = String To Byte Array(string=w137) -> (unsigned byte array=w136:u8[])
          n72 = Index Array(array=w144, index=w140) -> (element=w143:refnum<visa-resource-name>)
          n73 = Concatenate Strings("GPIB" ("string"), w162, "::" ("string"), w159, "::INSTR" ("string")) -> (w157:string)
          n74 = Index Array(array=w136, index=0) -> (element=w134:u8)
          n75 = VISA Open(error in (no error)=w142, VISA resource name=w157) -> (VISA resource name=w156:refnum<visa-resource-name>, error out=w155:errorcluster)  [unwired: 3 out]
          n76 = VISA Clear(VISA resource name=w156, error in (no error)=w155) -> (VISA resource name out=w146:refnum<visa-resource-name>, error out=w148:errorcluster)
          n77 = VISA Write(VISA resource name=w146, write buffer="xxx\n", error in (no error)=w148) -> (VISA resource name out=w145:refnum<visa-resource-name>, error out=w147:errorcluster)  [unwired: 1 out]
          n78 = property class="Instr"(reference=w145, "General Settings:Timeout Value"=w153) -> (reference out=w152:refnum<visa-resource-name>)  [unwired: 1 in, 1 out]
          n79 = property class="Instr"(reference=w152, "Message Based Settings:Termination Character Enable"=TRUE, "Message Based Settings:Termination Character"=w134) -> (reference out=w151:refnum<visa-resource-name>)  [unwired: 1 in, 1 out]
          n80 = Unbundle By Name(w147) -> ("status"=w141:bool, "code"=w154:i32)
        }
        frame 2 {
          # "Initialize DLL comm."
          n81 = Unbundle By Name(w179) -> ("DLL for Device"=w188:T6)
          n82 = case shown="17" w188 {
            tunnel: ["C843_GCS_DLL.dll" "C844_GCS_DLL.dll" "E7XX_GCS_DLL.dll" "C843_PM_GCS_DLL.dll" "C865_GCS_DLL.dll" "E7XX_GCS_DLL.dll" "PI_Mercury_GCS_DLL.dll" "PI_GCS2_DLL.dll" "PI_GCS2_DLL.dll" "C866_GCS_DLL.dll" "PI_GCS2_DLL.dll" "PI_GCS2_DLL.dll" "PI_GCS2_DLL.dll" "PI_GCS2_DLL.dll" "PI_GCS2_DLL.dll" "E816_DLL.dll" "PI_GCS2_DLL.dll" "PI_GCS2_DLL.dll" "PI_HydraPollux_GCS2_DLL.dll"] -> w189
            tunnel: ["C843_" "C844_" "E7XX_" "C843_PM_" "C865_" "E7XX_" "Mercury_" "PI_" "PI_" "C866_" "PI_" "PI_" "PI_" "PI_" "PI_" "E816_" "PI_" "PI_" "Hydra_"] -> w190
            frame 0, Default {
              # "C-843"
            }
            frame 1 {
              # "C-844"
            }
            frame 2 {
              # "E-710"
            }
            frame 3 {
              # "C-843.PM"
            }
            frame 4 {
              # "C-865"
            }
            frame 5 {
              # "E-761"
            }
            frame 6 {
              # "Mercury"
            }
            frame 7 {
              # "E-755"
            }
            frame 8 {
              # "E-753"
            }
            frame 9 {
              # "C-866"
            }
            frame 10 {
              # "E-712"
            }
            frame 11 {
              # "E-725"
            }
            frame 12 {
              # "E-861"
            }
            frame 13 {
              # "C-867"
            }
            frame 14 {
              # "E-517"
            }
            frame 15 {
              # "E-816.USB"
            }
            frame 16 {
              # "E-709"
            }
            frame 17 {
              # "PI_GCS2_DLL"
            }
            frame 18 {
              # "Hydra_Pollux"
            }
          }
          n83 = call "GCSTranslator DLL Functions.vi"("System no."=w176, "Function"=T11."DefineSystem", "String input"=w189, "error in"=w187, "String input 2"=w190) -> ("DLL I32 Return value"=w180:i32, "error out"=w181:errorcluster)  [unwired: 2 in, 11 out]
          n84 = Equal?(x=w180, y=-1) -> (x = y?=w184:bool)
          n85 = case shown="False" w184 {
            tunnel: w176 -> [w200 w361]
            tunnel: [w196 w360] -> w185
            tunnel: [w195 100 ("code")] -> w183
            tunnel: [w194 w358] -> w182
            tunnel: w181 -> [w198 w358]
            tunnel: w180 -> [w199 _]
            tunnel: w179 -> [w197 _]
            tunnel: [w193 TRUE] -> w178
            tunnel: w175 -> [w192 _]
            frame False {
              n86 = stacked-sequence {
                seq-local: [w202 _ _] -> [_ _ w226]
                tunnel: w200 -> [w205 w213 w222]
                tunnel: w199 -> [_ w212 _]
                tunnel: w198 -> [w204 _ _]
                tunnel: w197 -> [_ _ w228]
                tunnel: [_ _ w219] -> w194
                tunnel: [_ w212 _] -> w196
                tunnel: [_ _ w220] -> w195
                tunnel: [_ _ w218] -> w193
                tunnel: w192 -> [_ _ w217]
                frame #0 {
                  n87 = call "GCSTranslator DLL Functions.vi"("System no."=w205, "Function"=T11."IsConnected", "error in"=w204) -> ("Boolean output"=w206:bool, "error out"=w203:errorcluster)  [unwired: 4 in, 11 out]
                  n88 = case shown="True" w206 {
                    tunnel: w205 -> [_ w211]
                    tunnel: w203 -> [w207 w210]
                    tunnel: [w207 w209] -> w202
                    frame False {
                    }
                    frame True {
                      n89 = call "GCSTranslator DLL Functions.vi"("System no."=w211, "Function"=T11."CloseConnection", "error in"=w210) -> ("error out"=w209:errorcluster)  [unwired: 4 in, 12 out]
                    }
                  }
                }
                frame #1 {
                  n90 = Decrement(x=w213) -> (x-1=w214:i32)
                  n91 = global read "Global1.vi" "DLL device ID's"() -> (w215:i32[])
                  n92 = Replace Array Subset(array=w215, new element=w212, index=w214) -> (w216:i32[])
                  n93 = global write "Global1.vi" "DLL device ID's"(w216) -> ()
                }
                frame #2 {
                  n94 = Unbundle By Name(w228) -> ("DLL Interface"=w227:T7)
                  n95 = case shown="4" w227 {
                    tunnel: w222 -> [w240 w245 w250 w255 w259 w262 w294 w326]
                    tunnel: w226 -> [w239 w244 w249 w254 w257 w264 w296 w328]
                    tunnel: [w238 w243 w248 w253 w260 w265 w297 w329] -> w224
                    tunnel: [w237 w242 w247 w252 w256 w263 w295 w327] -> w221
                    tunnel: w217 -> [_ _ _ _ _ w261 w293 w325]
                    frame 0, Default {
                      # "RS-232"
                      n96 = call "GCSTranslator DLL Functions.vi"("System no."=w240, "Function"=T11."ConnectRS232", "error in"=w239) -> ("DLL I32 Return value"=w238:i32, "error out"=w237:errorcluster)  [unwired: 4 in, 11 out]
                    }
                    frame 1 {
                      # "GPIB"
                      n97 = call "GCSTranslator DLL Functions.vi"("System no."=w245, "Function"=T11."ConnectNIgpib", "error in"=w244) -> ("DLL I32 Return value"=w243:i32, "error out"=w242:errorcluster)  [unwired: 4 in, 11 out]
                    }
                    frame 2 {
                      # "Board"
                      n98 = call "GCSTranslator DLL Functions.vi"("System no."=w250, "Function"=T11."ConnectPciBoard", "error in"=w249) -> ("DLL I32 Return value"=w248:i32, "error out"=w247:errorcluster)  [unwired: 4 in, 11 out]
                    }
                    frame 3 {
                      # "TCP-IP"
                      n99 = call "GCSTranslator DLL Functions.vi"("System no."=w255, "Function"=T11."ConnectTCPIP", "error in"=w254) -> ("DLL I32 Return value"=w253:i32, "error out"=w252:errorcluster)  [unwired: 4 in, 11 out]
                    }
                    frame 4 {
                      # "USB"
                      n100 = call "GCSTranslator DLL Functions.vi"("System no."=w259, "Function"=T12."ConnectUSB", "error in"=w257) -> ("DLL I32 Return value"=w260:i32, "error out"=w256:errorcluster)  [unwired: 4 in, 11 out]
                    }
                    frame 5 {
                      # "RS232 DaisyChain"
                      n101 = case shown="False" w261 {
                        tunnel: [w266 w284] -> w265
                        tunnel: w264 -> [w271 w292]
                        tunnel: [w267 w287] -> w263
                        tunnel: w262 -> [w269 w286]
                        frame False {
                          n102 = call "Is DaisyChain open.vi"("System no."=w269, "error in"=w271) -> ("DC open?"=w270:bool, "error out"=w268:errorcluster)  [unwired: 16 out]
                          n103 = case shown="True" w270 {
                            tunnel: w269 -> [w276 w280]
                            tunnel: w268 -> [w274 w277]
                            tunnel: [w273 w282] -> w267
                            tunnel: [w272 w281] -> w266
                            frame True {
                              n104 = call "GCSTranslator DLL Functions.vi"("System no."=w276, "Function"=T13."ConnectDaisyChainDevice", "error in"=w274) -> ("DLL I32 Return value"=w272:i32, "error out"=w273:errorcluster)  [unwired: 4 in, 11 out]
                            }
                            frame False {
                              n105 = call "GCSTranslator DLL Functions.vi"("System no."=w280, "Function"=T13."OpenRS232DaisyChain", "error in"=w277) -> ("error out"=w278:errorcluster)  [unwired: 4 in, 12 out]
                              n106 = call "GCSTranslator DLL Functions.vi"("System no."=w280, "Function"=T13."ConnectDaisyChainDevice", "error in"=w278) -> ("DLL I32 Return value"=w281:i32, "error out"=w282:errorcluster)  [unwired: 4 in, 11 out]
                            }
                          }
                        }
                        frame True {
                          n107 = call "GCSTranslator DLL Functions.vi"("System no."=w286, "Function"=T13."CloseDaisyChain", "error in"=w292) -> ("error out"=w290:errorcluster)  [unwired: 4 in, 12 out]
                          n108 = call "GCSTranslator DLL Functions.vi"("System no."=w286, "Function"=T13."OpenRS232DaisyChain", "error in"=w290) -> ("error out"=w288:errorcluster)  [unwired: 4 in, 12 out]
                          n109 = call "GCSTranslator DLL Functions.vi"("System no."=w286, "Function"=T13."ConnectDaisyChainDevice", "error in"=w288) -> ("DLL I32 Return value"=w284:i32, "error out"=w287:errorcluster)  [unwired: 4 in, 11 out]
                        }
                      }
                    }
                    frame 6 {
                      # "USB DaisyChain"
                      n110 = case shown="True" w293 {
                        tunnel: [w298 w317] -> w297
                        tunnel: w296 -> [w303 w324]
                        tunnel: [w299 w320] -> w295
                        tunnel: w294 -> [w301 w319]
                        frame False {
                          n111 = call "Is DaisyChain open.vi"("System no."=w301, "error in"=w303) -> ("DC open?"=w302:bool, "error out"=w300:errorcluster)  [unwired: 16 out]
                          n112 = case shown="True" w302 {
                            tunnel: w301 -> [w308 w313]
                            tunnel: w300 -> [w306 w311]
                            tunnel: [w305 w309] -> w299
                            tunnel: [w304 w314] -> w298
                            frame True {
                              n113 = call "GCSTranslator DLL Functions.vi"("System no."=w308, "Function"=T13."ConnectDaisyChainDevice", "error in"=w306) -> ("DLL I32 Return value"=w304:i32, "error out"=w305:errorcluster)  [unwired: 4 in, 11 out]
                            }
                            frame False {
                              n114 = call "GCSTranslator DLL Functions.vi"("System no."=w313, "Function"=T14."OpenUSBDaisyChain", "error in"=w311) -> ("error out"=w312:errorcluster)  [unwired: 4 in, 12 out]
                              n115 = call "GCSTranslator DLL Functions.vi"("System no."=w313, "Function"=T13."ConnectDaisyChainDevice", "error in"=w312) -> ("DLL I32 Return value"=w314:i32, "error out"=w309:errorcluster)  [unwired: 4 in, 11 out]
                            }
                          }
                        }
                        frame True {
                          n116 = call "GCSTranslator DLL Functions.vi"("System no."=w319, "Function"=T13."CloseDaisyChain", "error in"=w324) -> ("error out"=w322:errorcluster)  [unwired: 4 in, 12 out]
                          n117 = call "GCSTranslator DLL Functions.vi"("System no."=w319, "Function"=T14."OpenUSBDaisyChain", "error in"=w322) -> ("error out"=w321:errorcluster)  [unwired: 4 in, 12 out]
                          n118 = call "GCSTranslator DLL Functions.vi"("System no."=w319, "Function"=T13."ConnectDaisyChainDevice", "error in"=w321) -> ("DLL I32 Return value"=w317:i32, "error out"=w320:errorcluster)  [unwired: 4 in, 11 out]
                        }
                      }
                    }
                    frame 7 {
                      # "TCPIP DaisyChain"
                      n119 = case shown="False" w325 {
                        tunnel: [w330 w349] -> w329
                        tunnel: w328 -> [w335 w356]
                        tunnel: [w331 w352] -> w327
                        tunnel: w326 -> [w333 w351]
                        frame False {
                          n120 = call "Is DaisyChain open.vi"("System no."=w333, "error in"=w335) -> ("DC open?"=w334:bool, "error out"=w332:errorcluster)  [unwired: 16 out]
                          n121 = case shown="True" w334 {
                            tunnel: w333 -> [w340 w346]
                            tunnel: w332 -> [w339 w344]
                            tunnel: [w338 w342] -> w331
                            tunnel: [w337 w347] -> w330
                            frame True {
                              n122 = call "GCSTranslator DLL Functions.vi"("System no."=w340, "Function"=T15."ConnectDaisyChainDevice", "error in"=w339) -> ("DLL I32 Return value"=w337:i32, "error out"=w338:errorcluster)  [unwired: 4 in, 11 out]
                            }
                            frame False {
                              n123 = call "GCSTranslator DLL Functions.vi"("System no."=w346, "Function"=T15."OpenTCPIPDaisyChain", "error in"=w344) -> ("error out"=w345:errorcluster)  [unwired: 4 in, 12 out]
                              n124 = call "GCSTranslator DLL Functions.vi"("System no."=w346, "Function"=T15."ConnectDaisyChainDevice", "error in"=w345) -> ("DLL I32 Return value"=w347:i32, "error out"=w342:errorcluster)  [unwired: 4 in, 11 out]
                            }
                          }
                        }
                        frame True {
                          n125 = call "GCSTranslator DLL Functions.vi"("System no."=w351, "Function"=T13."CloseDaisyChain", "error in"=w356) -> ("error out"=w354:errorcluster)  [unwired: 4 in, 12 out]
                          n126 = call "GCSTranslator DLL Functions.vi"("System no."=w351, "Function"=T15."OpenTCPIPDaisyChain", "error in"=w354) -> ("error out"=w353:errorcluster)  [unwired: 4 in, 12 out]
                          n127 = call "GCSTranslator DLL Functions.vi"("System no."=w351, "Function"=T13."ConnectDaisyChainDevice", "error in"=w353) -> ("DLL I32 Return value"=w349:i32, "error out"=w352:errorcluster)  [unwired: 4 in, 11 out]
                        }
                      }
                    }
                  }
                  n128 = Equal?(x=w224, y=-1) -> (x = y?=w223:bool)
                  n129 = case shown="False" w223 {
                    tunnel: w222 -> [_ w235]
                    tunnel: w221 -> [w230 w234]
                    tunnel: [w230 w233] -> w219
                    tunnel: [w229 w232] -> w220
                    frame False {
                      n130 = Unbundle By Name(w230) -> ("code"=w229:i32)
                    }
                    frame True {
                      # "Error!"
                      n131 = call "GCSTranslator DLL Functions.vi"("System no."=w235, "Function"=T11."GetError", "error in"=w234) -> ("error out"=w233:errorcluster)  [unwired: 4 in, 12 out]
                      n132 = Unbundle By Name(w233) -> ("code"=w232:i32)
                    }
                  }
                  n133 = Unbundle By Name(w219) -> ("status"=w218:bool)
                }
              }
            }
            frame True {
              # "Error: do not change ID's"
              n134 = global read "Global1.vi" "DLL device ID's"() -> (w363:i32[])
              n135 = Decrement(x=w361) -> (x-1=w362:i32)
              n136 = Index Array(array=w363, index=w362) -> (element=w360:i32)
            }
          }
        }
        frame 3 {
          w427 = "::" ("string")
          # "Initialize TCP/IP comm."
          n137 = flat-sequence {
            tunnel: w408 -> [w441]
            tunnel: w404 -> [w440]
            tunnel: [w440] -> w403
            tunnel: [w439] -> w402
            tunnel: [w443] -> w407
            tunnel: w403 -> [w443]
            tunnel: w402 -> [_]
            frame #0 {
              n138 = VISA Close(VISA resource name=w441, error in (no error)=w440) -> (error out=w439:errorcluster)
            }
            frame #1 {
              n139 = Wait (ms)(milliseconds to wait=u32 50) -> ()  [unwired: 1 out]
            }
          }
          n140 = Unbundle By Name(w425) -> ("Timeout"=w424:i32)
          n141 = Unbundle By Name(w434) -> ("Host address/name"=w430:string, "Port"=w429:i32, "Board"=w432:i32)
          n142 = case shown="\"LF\", Default" w414 {
            tunnel: ["\n" "\r" "\r" "\n"] -> w413
            frame "LF", Default {
            }
            frame "CR" {
            }
            frame "LFCR" {
            }
            frame "CRLF" {
            }
          }
          n143 = global read "Global1.vi" "VISA Resource name"() -> (w409:refnum<visa-resource-name>[])
          n144 = Index Array(array=w409, index=w405) -> (element=w408:refnum<visa-resource-name>)
          n145 = String To Byte Array(string=w413) -> (unsigned byte array=w412:u8[])
          n146 = Index Array(array=w412, index=0) -> (element=w410:u8)
          n147 = Number To Decimal String(number=w429) -> (decimal integer string=w428:string)  [unwired: 1 out]
          n148 = Not Equal To 0?(x=w432) -> (x != 0?=w433:bool)
          n149 = case shown="True" w433 {
            tunnel: w432 -> [_ w450]
            tunnel: ["" w449] -> w431
            frame False {
            }
            frame True {
              n150 = Number To Decimal String(number=w450) -> (decimal integer string=w449:string)  [unwired: 1 out]
            }
          }
          n151 = Concatenate Strings("TCPIP" ("string"), w431, w427, w430, w427, w428, "::SOCKET" ("string")) -> (w437:string)
          n152 = VISA Open(error in (no error)=w407, VISA resource name=w437) -> (VISA resource name=w436:refnum<visa-resource-name>, error out=w435:errorcluster)  [unwired: 3 out]
          n153 = VISA Clear(VISA resource name=w436, error in (no error)=w435) -> (VISA resource name out=w420:refnum<visa-resource-name>, error out=w418:errorcluster)
          n154 = VISA Write(VISA resource name=w420, write buffer="xxx\n", error in (no error)=w418) -> (VISA resource name out=w419:refnum<visa-resource-name>, error out=w416:errorcluster)  [unwired: 1 out]
          n155 = property class="Instr"(reference=w419, "General Settings:Timeout Value"=w424, "Message Based Settings:Termination Character Enable"=TRUE, "Message Based Settings:Termination Character"=w410) -> (reference out=w423:refnum<visa-resource-name>)  [unwired: 1 in, 1 out]
          n156 = Unbundle By Name(w416) -> ("status"=w406:bool, "code"=w422:i32)
        }
        frame 4 {
          # "Initialize USB comm."
        }
        frame 5 {
          # "Initialize Analog comm."
        }
        frame 6 {
          # "Initialize DLL communication"
          n157 = Unbundle By Name(w467) -> ("DLL for Device"=w469:T6)
          n158 = case shown="0, Default" w469 {
            tunnel: w467 -> [w478 w522 w566 w627 w671 w739 w792]
            tunnel: [w473 w517 w558 w619 w664 w734 w785] -> w462
            tunnel: [w471 w515 w559 w620 w663 w733 w784] -> w468
            tunnel: w461 -> [w476 w520 w563 w624 w668 w728 w790]
            tunnel: [w475 w519 w564 w625 w669 w737 w789] -> w466
            tunnel: w464 -> [w474 w518 w562 w623 w667 _ w788]
            tunnel: w461 -> [w472 w516 w560 w622 w665 w735 w786]
            tunnel: [w470 w514 w561 w621 w666 w736 w787] -> w463
            frame 0, Default {
              # "C-843"
              n159 = Unbundle By Name(w478) -> ("DLL Interface"=w477:T7)
              n160 = case shown="2" w477 {
                tunnel: [TRUE TRUE w498] -> w473
                tunnel: [100 100 w497] -> w471
                tunnel: w476 -> [_ _ w494]
                tunnel: [w488 w491 w495] -> w475
                tunnel: w474 -> [w488 w491 _]
                frame 0, Default {
                  # "not available for C-843"
                  # "RS-232"
                }
                frame 1 {
                  # "not available for C-843"
                  # "GPIB"
                }
                frame 2 {
                  # "Board"
                  n161 = call "GCSTranslator DLL Functions.vi"("System no."=w494, "Function"=T16."C843_IsDLLAvailable") -> ("Boolean output"=w500:bool, "error out"=w499:errorcluster)  [unwired: 5 in, 11 out]
                  n162 = case shown="True" w500 {
                    tunnel: [TRUE w513] -> w498
                    tunnel: w494 -> [_ w512]
                    tunnel: [w502 w510] -> w497
                    tunnel: w499 -> [w501 w509]
                    tunnel: [w501 w507] -> w495
                    frame False {
                      n163 = case shown="Error" w501 {
                        tunnel: [-33 ("DLL I32 Return value") w505] -> w502
                        tunnel: w501 -> [_ w506]
                        frame No Error {
                        }
                        frame Error {
                          n164 = Unbundle By Name(w506) -> ("code"=w505:i32)
                        }
                      }
                    }
                    frame True {
                      n165 = call "Close connection if open.vi"("System no."=w512, "error in"=w509) -> ("error out"=w511:errorcluster)  [unwired: 1 in, 16 out]
                      n166 = call "GCSTranslator DLL Functions.vi"("System no."=w512, "Function"=T16."C843_Connect", "error in"=w511) -> ("DLL I32 Return value"=w510:i32, "error out"=w507:errorcluster)  [unwired: 4 in, 11 out]
                      n167 = Less Than 0?(x=w510) -> (x < 0?=w513:bool)
                    }
                  }
                }
              }
              n168 = case shown="True" w473 {
                tunnel: w471 -> [w479 _]
                tunnel: w472 -> [w483 w485]
                tunnel: [w479 w484] -> w470
                frame False {
                  n169 = Decrement(x=w483) -> (x-1=w482:i32)
                  n170 = global read "Global1.vi" "DLL device ID's"() -> (w481:i32[])
                  n171 = Replace Array Subset(array=w481, new element=w479, index=w482) -> (w480:i32[])
                  n172 = global write "Global1.vi" "DLL device ID's"(w480) -> ()
                }
                frame True {
                  # "Error: do not change ID's"
                  n173 = global read "Global1.vi" "DLL device ID's"() -> (w487:i32[])
                  n174 = Decrement(x=w485) -> (x-1=w486:i32)
                  n175 = Index Array(array=w487, index=w486) -> (element=w484:i32)
                }
              }
            }
            frame 5 {
              # "E-761"
              n176 = Unbundle By Name(w522) -> ("DLL Interface"=w521:T7)
              n177 = case shown="2" w521 {
                tunnel: [TRUE TRUE w542] -> w517
                tunnel: [100 100 w541] -> w515
                tunnel: w520 -> [_ _ w539]
                tunnel: [w532 w535 w540] -> w519
                tunnel: w518 -> [w532 w535 _]
                frame 0, Default {
                  # "not available for E-761"
                  # "RS-232"
                }
                frame 1 {
                  # "Not available for E-761"
                  # "GPIB"
                }
                frame 2 {
                  # "Board"
                  n178 = call "GCSTranslator DLL Functions.vi"("System no."=w539, "Function"=T11."E710_IsDLLAvailable") -> ("Boolean output"=w544:bool, "error out"=w543:errorcluster)  [unwired: 5 in, 11 out]
                  n179 = case shown="True" w544 {
                    tunnel: [TRUE w557] -> w542
                    tunnel: w539 -> [_ w556]
                    tunnel: [w546 w554] -> w541
                    tunnel: w543 -> [w545 w553]
                    tunnel: [w545 w552] -> w540
                    frame False {
                      n180 = case shown="Error" w545 {
                        tunnel: [-33 ("DLL I32 Return value") w549] -> w546
                        tunnel: w545 -> [_ w550]
                        frame No Error {
                        }
                        frame Error {
                          n181 = Unbundle By Name(w550) -> ("code"=w549:i32)
                        }
                      }
                    }
                    frame True {
                      n182 = call "Close connection if open.vi"("System no."=w556, "error in"=w553) -> ("error out"=w555:errorcluster)  [unwired: 1 in, 16 out]
                      n183 = call "GCSTranslator DLL Functions.vi"("System no."=w556, "Function"=T11."E761_ConnectPciBoard", "error in"=w555) -> ("DLL I32 Return value"=w554:i32, "error out"=w552:errorcluster)  [unwired: 4 in, 11 out]
                      n184 = Less Than 0?(x=w554) -> (x < 0?=w557:bool)
                    }
                  }
                }
              }
              n185 = case shown="True" w517 {
                tunnel: w515 -> [w523 _]
                tunnel: w516 -> [w527 w529]
                tunnel: [w523 w528] -> w514
                frame False {
                  n186 = Decrement(x=w527) -> (x-1=w526:i32)
                  n187 = global read "Global1.vi" "DLL device ID's"() -> (w525:i32[])
                  n188 = Replace Array Subset(array=w525, new element=w523, index=w526) -> (w524:i32[])
                  n189 = global write "Global1.vi" "DLL device ID's"(w524) -> ()
                }
                frame True {
                  # "Error: do not change ID's"
                  n190 = global read "Global1.vi" "DLL device ID's"() -> (w531:i32[])
                  n191 = Decrement(x=w529) -> (x-1=w530:i32)
                  n192 = Index Array(array=w531, index=w530) -> (element=w528:i32)
                }
              }
            }
            frame 1 {
              # "C-844"
              n193 = Unbundle By Name(w566) -> ("DLL Interface"=w565:T7)
              n194 = case shown="0, Default" w565 {
                tunnel: [w582 w602 TRUE] -> w558
                tunnel: [w581 w601 100] -> w559
                tunnel: w563 -> [w576 w596 _]
                tunnel: [w577 w597 w616] -> w564
                tunnel: w562 -> [_ _ w616]
                frame 0, Default {
                  # "RS-232"
                  n195 = call "GCSTranslator DLL Functions.vi"("System no."=w576, "Function"=T17."C844_IsDLLAvailable") -> ("Boolean output"=w579:bool, "error out"=w578:errorcluster)  [unwired: 5 in, 11 out]
                  n196 = case shown="False" w579 {
                    tunnel: [TRUE w595] -> w582
                    tunnel: w576 -> [_ w594]
                    tunnel: [w584 w592] -> w581
                    tunnel: w578 -> [w583 w590]
                    tunnel: [w583 w589] -> w577
                    frame False {
                      n197 = case shown="No Error" w583 {
                        tunnel: [-33 ("DLL I32 Return value") w587] -> w584
                        tunnel: w583 -> [_ w588]
                        frame No Error {
                        }
                        frame Error {
                          n198 = Unbundle By Name(w588) -> ("code"=w587:i32)
                        }
                      }
                    }
                    frame True {
                      # "RS-232"
                      n199 = call "Close connection if open.vi"("System no."=w594, "error in"=w590) -> ("error out"=w593:errorcluster)  [unwired: 1 in, 16 out]
                      n200 = call "GCSTranslator DLL Functions.vi"("System no."=w594, "Function"=T17."C844_ConnectRS232", "error in"=w593) -> ("DLL I32 Return value"=w592:i32, "error out"=w589:errorcluster)  [unwired: 4 in, 11 out]
                      n201 = Less Than 0?(x=w592) -> (x < 0?=w595:bool)
                    }
                  }
                }
                frame 1 {
                  # "GPIB"
                  n202 = call "GCSTranslator DLL Functions.vi"("System no."=w596, "Function"=T17."C844_IsDLLAvailable") -> ("Boolean output"=w600:bool, "error out"=w599:errorcluster)  [unwired: 5 in, 11 out]
                  n203 = case shown="False" w600 {
                    tunnel: [TRUE w615] -> w602
                    tunnel: w596 -> [_ w614]
                    tunnel: [w604 w612] -> w601
                    tunnel: w599 -> [w603 w610]
                    tunnel: [w603 w609] -> w597
                    frame False {
                      n204 = case shown="No Error" w603 {
                        tunnel: [-33 ("DLL I32 Return value") w607] -> w604
                        tunnel: w603 -> [_ w608]
                        frame No Error {
                        }
                        frame Error {
                          n205 = Unbundle By Name(w608) -> ("code"=w607:i32)
                        }
                      }
                    }
                    frame True {
                      n206 = call "Close connection if open.vi"("System no."=w614, "error in"=w610) -> ("error out"=w613:errorcluster)  [unwired: 1 in, 16 out]
                      n207 = call "GCSTranslator DLL Functions.vi"("System no."=w614, "Function"=T17."C844_ConnectNIgpib", "error in"=w613) -> ("DLL I32 Return value"=w612:i32, "error out"=w609:errorcluster)  [unwired: 4 in, 11 out]
                      n208 = Less Than 0?(x=w612) -> (x < 0?=w615:bool)
                    }
                  }
                }
                frame 2 {
                  # "not available for C-844"
                  # "Board"
                }
              }
              n209 = case shown="False" w558 {
                tunnel: w559 -> [w567 _]
                tunnel: w560 -> [w571 w573]
                tunnel: [w567 w572] -> w561
                frame False {
                  n210 = Decrement(x=w571) -> (x-1=w570:i32)
                  n211 = global read "Global1.vi" "DLL device ID's"() -> (w569:i32[])
                  n212 = Replace Array Subset(array=w569, new element=w567, index=w570) -> (w568:i32[])
                  n213 = global write "Global1.vi" "DLL device ID's"(w568) -> ()
                }
                frame True {
                  # "Error: do not change ID's"
                  n214 = global read "Global1.vi" "DLL device ID's"() -> (w575:i32[])
                  n215 = Decrement(x=w573) -> (x-1=w574:i32)
                  n216 = Index Array(array=w575, index=w574) -> (element=w572:i32)
                }
              }
            }
            frame 4 {
              # "C-865"
              n217 = Unbundle By Name(w627) -> ("DLL Interface"=w626:T7)
              n218 = case shown="0, Default" w626 {
                tunnel: [w643 TRUE TRUE] -> w619
                tunnel: [w642 100 100] -> w620
                tunnel: w624 -> [w637 _ _]
                tunnel: [w638 w657 w660] -> w625
                tunnel: w623 -> [_ w657 w660]
                frame 0, Default {
                  # "RS-232"
                  n219 = call "GCSTranslator DLL Functions.vi"("System no."=w637, "Function"=T18."C865_IsDLLAvailable") -> ("Boolean output"=w640:bool, "error out"=w639:errorcluster)  [unwired: 5 in, 11 out]
                  n220 = case shown="True" w640 {
                    tunnel: [TRUE w656] -> w643
                    tunnel: w637 -> [_ w655]
                    tunnel: [w645 w653] -> w642
                    tunnel: w639 -> [w644 w652]
                    tunnel: [w644 w651] -> w638
                    frame False {
                      n221 = case shown="No Error" w644 {
                        tunnel: [-33 ("DLL I32 Return value") w648] -> w645
                        tunnel: w644 -> [_ w649]
                        frame No Error {
                        }
                        frame Error {
                          n222 = Unbundle By Name(w649) -> ("code"=w648:i32)
                        }
                      }
                    }
                    frame True {
                      # "RS-232"
                      n223 = call "Close connection if open.vi"("System no."=w655, "error in"=w652) -> ("error out"=w654:errorcluster)  [unwired: 1 in, 16 out]
                      n224 = call "GCSTranslator DLL Functions.vi"("System no."=w655, "Function"=T18."C865_ConnectRS232", "error in"=w654) -> ("DLL I32 Return value"=w653:i32, "error out"=w651:errorcluster)  [unwired: 4 in, 11 out]
                      n225 = Less Than 0?(x=w653) -> (x < 0?=w656:bool)
                    }
                  }
                }
                frame 2 {
                  # "not available for C-865"
                  # "Board"
                }
                frame 1 {
                  # "not available for C-865"
                  # "GPIB"
                }
              }
              n226 = case shown="False" w619 {
                tunnel: w620 -> [w628 _]
                tunnel: w622 -> [w632 w634]
                tunnel: [w628 w633] -> w621
                frame False {
                  n227 = Decrement(x=w632) -> (x-1=w631:i32)
                  n228 = global read "Global1.vi" "DLL device ID's"() -> (w630:i32[])
                  n229 = Replace Array Subset(array=w630, new element=w628, index=w631) -> (w629:i32[])
                  n230 = global write "Global1.vi" "DLL device ID's"(w629) -> ()
                }
                frame True {
                  # "Error: do not change ID's"
                  n231 = global read "Global1.vi" "DLL device ID's"() -> (w636:i32[])
                  n232 = Decrement(x=w634) -> (x-1=w635:i32)
                  n233 = Index Array(array=w636, index=w635) -> (element=w633:i32)
                }
              }
            }
            frame 2 {
              # "E-710"
              n234 = Unbundle By Name(w671) -> ("DLL Interface"=w670:T7)
              n235 = case shown="0, Default" w670 {
                tunnel: [w688 w708 TRUE] -> w664
                tunnel: [w687 w707 100] -> w663
                tunnel: w668 -> [w683 w702 _]
                tunnel: [w685 w704 w722] -> w669
                tunnel: w667 -> [w682 _ w722]
                frame 0, Default {
                  # "RS-232"
                  n236 = call "GCSTranslator DLL Functions.vi"("System no."=w683, "Function"=T19."E710_IsDLLAvailable", "error in"=w682) -> ("Boolean output"=w681:bool, "error out"=w686:errorcluster)  [unwired: 4 in, 11 out]
                  n237 = case shown="True" w681 {
                    tunnel: [TRUE w701] -> w688
                    tunnel: w683 -> [_ w700]
                    tunnel: [w690 w698] -> w687
                    tunnel: w686 -> [w689 w697]
                    tunnel: [w689 w696] -> w685
                    frame False {
                      n238 = case shown="No Error" w689 {
                        tunnel: [-33 ("DLL I32 Return value") w693] -> w690
                        tunnel: w689 -> [_ w694]
                        frame No Error {
                        }
                        frame Error {
                          n239 = Unbundle By Name(w694) -> ("code"=w693:i32)
                        }
                      }
                    }
                    frame True {
                      # "RS-232"
                      n240 = call "Close connection if open.vi"("System no."=w700, "error in"=w697) -> ("error out"=w699:errorcluster)  [unwired: 1 in, 16 out]
                      n241 = call "GCSTranslator DLL Functions.vi"("System no."=w700, "Function"=T19."E710_ConnectRS232", "error in"=w699) -> ("DLL I32 Return value"=w698:i32, "error out"=w696:errorcluster)  [unwired: 4 in, 11 out]
                      n242 = Less Than 0?(x=w698) -> (x < 0?=w701:bool)
                    }
                  }
                }
                frame 1 {
                  # "GPIB"
                  n243 = call "GCSTranslator DLL Functions.vi"("System no."=w702, "Function"=T19."E710_IsDLLAvailable") -> ("Boolean output"=w706:bool, "error out"=w705:errorcluster)  [unwired: 5 in, 11 out]
                  n244 = case shown="True" w706 {
                    tunnel: [TRUE w721] -> w708
                    tunnel: w702 -> [_ w720]
                    tunnel: [w710 w718] -> w707
                    tunnel: w705 -> [w709 w717]
                    tunnel: [w709 w716] -> w704
                    frame False {
                      n245 = case shown="No Error" w709 {
                        tunnel: [-33 ("DLL I32 Return value") w713] -> w710
                        tunnel: w709 -> [_ w714]
                        frame No Error {
                        }
                        frame Error {
                          n246 = Unbundle By Name(w714) -> ("code"=w713:i32)
                        }
                      }
                    }
                    frame True {
                      n247 = call "Close connection if open.vi"("System no."=w720, "error in"=w717) -> ("error out"=w719:errorcluster)  [unwired: 1 in, 16 out]
                      n248 = call "GCSTranslator DLL Functions.vi"("System no."=w720, "Function"=T19."E710_ConnectNIgpib", "error in"=w719) -> ("DLL I32 Return value"=w718:i32, "error out"=w716:errorcluster)  [unwired: 4 in, 11 out]
                      n249 = Less Than 0?(x=w718) -> (x < 0?=w721:bool)
                    }
                  }
                }
                frame 2 {
                  # "not available for E-710"
                  # "Board"
                }
              }
              n250 = case shown="True" w664 {
                tunnel: w663 -> [w672 _]
                tunnel: w665 -> [w676 w678]
                tunnel: [w672 w677] -> w666
                frame False {
                  n251 = Decrement(x=w676) -> (x-1=w675:i32)
                  n252 = global read "Global1.vi" "DLL device ID's"() -> (w674:i32[])
                  n253 = Replace Array Subset(array=w674, new element=w672, index=w675) -> (w673:i32[])
                  n254 = global write "Global1.vi" "DLL device ID's"(w673) -> ()
                }
                frame True {
                  # "Error: do not change ID's"
                  n255 = global read "Global1.vi" "DLL device ID's"() -> (w680:i32[])
                  n256 = Decrement(x=w678) -> (x-1=w679:i32)
                  n257 = Index Array(array=w680, index=w679) -> (element=w677:i32)
                }
              }
            }
            frame 6 {
              # "Mercury"
              n258 = Unbundle By Name(w739) -> ("DLL Interface"=w738:T7)
              n259 = call "GCSTranslator DLL Functions.vi"("System no."=w728, "Function"=T11."DefineSystem", "String input"="PI_Mercury_GCS_DLL.dll", "String input 2"="Mercury_") -> ("DLL I32 Return value"=w727:i32, "error out"=w730:errorcluster)  [unwired: 3 in, 11 out]
              n260 = Equal?(x=w727, y=-1) -> (x = y?=w726:bool)
              n261 = case shown="True" w726 {
                tunnel: w738 -> [w745 _]
                tunnel: [w744 w772] -> w737
                tunnel: [w743 TRUE] -> w734
                tunnel: [w742 -1 ("DLL I32 Return value")] -> w733
                tunnel: w730 -> [w741 w772]
                tunnel: w728 -> [w740 _]
                frame False {
                  n262 = case shown="0, Default" w745 {
                    tunnel: [w748 TRUE ("status") TRUE] -> w743
                    tunnel: [w747 100 ("code") 100] -> w742
                    tunnel: w740 -> [w750 _ _]
                    tunnel: [w746 w766 w769] -> w744
                    tunnel: w741 -> [w749 w766 w769]
                    frame 0, Default {
                      # "RS-232"
                      n263 = call "Close connection if open.vi"("System no."=w750, "error in"=w749) -> ("error out"=w751:errorcluster)  [unwired: 1 in, 16 out]
                      n264 = call "GCSTranslator DLL Functions.vi"("System no."=w750, "Function"=T11."ConnectRS232", "error in"=w751) -> ("DLL I32 Return value"=w755:i32, "error out"=w754:errorcluster)  [unwired: 4 in, 11 out]
                      n265 = Equal?(x=w755, y=-1) -> (x = y?=w753:bool)
                      n266 = case shown="True" w753 {
                        tunnel: w750 -> [_ w765]
                        tunnel: w754 -> [w757 w764]
                        tunnel: [w757 w763] -> w746
                        tunnel: [w758 w762] -> w747
                        tunnel: [w759 w761] -> w748
                        frame False {
                          n267 = Unbundle By Name(w757) -> ("status"=w759:bool, "code"=w758:i32)
                        }
                        frame True {
                          n268 = call "GCSTranslator DLL Functions.vi"("System no."=w765, "Function"=T11."GetError", "error in"=w764) -> ("error out"=w763:errorcluster)  [unwired: 4 in, 12 out]
                          n269 = Unbundle By Name(w763) -> ("status"=w761:bool, "code"=w762:i32)
                        }
                      }
                    }
                    frame 1 {
                      # "not available for Mercury"
                      # "GPIB"
                    }
                    frame 2 {
                      # "not available for Mercury"
                      # "Board"
                    }
                  }
                }
                frame True {
                }
              }
              n270 = case shown="False" w734 {
                tunnel: w733 -> [w775 _]
                tunnel: w735 -> [w779 w781]
                tunnel: [w775 w780] -> w736
                frame False {
                  n271 = Decrement(x=w779) -> (x-1=w778:i32)
                  n272 = global read "Global1.vi" "DLL device ID's"() -> (w777:i32[])
                  n273 = Replace Array Subset(array=w777, new element=w775, index=w778) -> (w776:i32[])
                  n274 = global write "Global1.vi" "DLL device ID's"(w776) -> ()
                }
                frame True {
                  # "Error: do not change ID's"
                  n275 = global read "Global1.vi" "DLL device ID's"() -> (w783:i32[])
                  n276 = Decrement(x=w781) -> (x-1=w782:i32)
                  n277 = Index Array(array=w783, index=w782) -> (element=w780:i32)
                }
              }
            }
            frame 3 {
              # "C-843.PM"
              n278 = Unbundle By Name(w792) -> ("DLL Interface"=w791:T7)
              n279 = case shown="2" w791 {
                tunnel: [TRUE TRUE w812] -> w785
                tunnel: [100 100 w811] -> w784
                tunnel: w790 -> [_ _ w809]
                tunnel: [w802 w805 w810] -> w789
                tunnel: w788 -> [w802 w805 _]
                frame 0, Default {
                  # "not available for C-843.PM"
                  # "RS-232"
                }
                frame 1 {
                  # "not available for C-843.PM"
                  # "GPIB"
                }
                frame 2 {
                  # "Board"
                  n280 = call "GCSTranslator DLL Functions.vi"("System no."=w809, "Function"=T20."C843_PM_IsDLLAvailable") -> ("Boolean output"=w814:bool, "error out"=w813:errorcluster)  [unwired: 5 in, 11 out]
                  n281 = case shown="True" w814 {
                    tunnel: [TRUE w827] -> w812
                    tunnel: w809 -> [_ w826]
                    tunnel: [w816 w824] -> w811
                    tunnel: w813 -> [w815 w823]
                    tunnel: [w815 w822] -> w810
                    frame False {
                      n282 = case shown="No Error" w815 {
                        tunnel: [-33 ("DLL I32 Return value") w819] -> w816
                        tunnel: w815 -> [_ w820]
                        frame No Error {
                        }
                        frame Error {
                          n283 = Unbundle By Name(w820) -> ("code"=w819:i32)
                        }
                      }
                    }
                    frame True {
                      n284 = call "Close connection if open.vi"("System no."=w826, "error in"=w823) -> ("error out"=w825:errorcluster)  [unwired: 1 in, 16 out]
                      n285 = call "GCSTranslator DLL Functions.vi"("System no."=w826, "Function"=T20."C843_PM_Connect", "error in"=w825) -> ("DLL I32 Return value"=w824:i32, "error out"=w822:errorcluster)  [unwired: 4 in, 11 out]
                      n286 = Less Than 0?(x=w824) -> (x < 0?=w827:bool)
                    }
                  }
                }
              }
              n287 = case shown="True" w785 {
                tunnel: w784 -> [w793 _]
                tunnel: w786 -> [w797 w799]
                tunnel: [w793 w798] -> w787
                frame False {
                  n288 = Decrement(x=w797) -> (x-1=w796:i32)
                  n289 = global read "Global1.vi" "DLL device ID's"() -> (w795:i32[])
                  n290 = Replace Array Subset(array=w795, new element=w793, index=w796) -> (w794:i32[])
                  n291 = global write "Global1.vi" "DLL device ID's"(w794) -> ()
                }
                frame True {
                  # "Error: do not change ID's"
                  n292 = global read "Global1.vi" "DLL device ID's"() -> (w801:i32[])
                  n293 = Decrement(x=w799) -> (x-1=w800:i32)
                  n294 = Index Array(array=w801, index=w800) -> (element=w798:i32)
                }
              }
            }
          }
        }
      }
      "DLL device ID" <- w20
      n295 = global read "Global1.vi" "VISA Resource name"() -> (w24:refnum<visa-resource-name>[])
      n296 = Replace Array Subset(array=w24, new element=w22, index=w11) -> (w23:refnum<visa-resource-name>[])
      n297 = global write "Global1.vi" "VISA Resource name"(w23) -> ()
      n298 = case shown="True" w12 {
        tunnel: w19 -> [_ w867]
        tunnel: w28 -> [w859 w860]
        tunnel: [w859 w864] -> w27
        frame False {
          # "no error"
        }
        frame True {
          n299 = Equal?(x=w867, y=100) -> (x = y?=w865:bool)
          n300 = case shown="False" w865 {
            tunnel: [w877 w904] -> w861
            tunnel: w867 -> [w869 w905]
            tunnel: [w868 w905] -> w862
            tunnel: w860 -> [_ _]
            frame False {
              n301 = Equal?(x=w869, y=-33) -> (x = y?=w884:bool)
              n302 = case shown="True" w884 {
                tunnel: ["" ("Substring") "error: a required DLL is not available. " ("Substring")] -> w883
                frame False {
                }
                frame True {
                }
              }
              n303 = Build Array(-1073807343 ("y"), -1073807202 ("y")) -> (w872:i32[])
              n304 = Equal?(x=w869, y=w872) -> (x = y?=w871:bool[])
              n305 = Build Array(-1073807343 ("y"), -1073807195 ("y")) -> (w890:i32[])
              n306 = Or Array Elements(Boolean array=w871) -> (logical OR=w870:bool)
              n307 = Equal?(x=w869, y=w890) -> (x = y?=w891:bool[])
              n308 = case shown="False" w870 {
                tunnel: ["" ("Substring") "error: Please check if NI VISA is installed  properly." ("Substring")] -> w875
                frame False {
                }
                frame True {
                }
              }
              n309 = Or Array Elements(Boolean array=w891) -> (logical OR=w887:bool)
              n310 = case shown="True" w887 {
                tunnel: ["" ("Substring") "error: Could not open connection.\nPossible reasons: \ninvalid host name, port or interface number,\ndevice or resource not present." ("Substring")] -> w886
                frame False {
                }
                frame True {
                }
              }
              n311 = Equal?(x=w869, y=-9) -> (x = y?=w881:bool)
              n312 = case shown="True" w881 {
                tunnel: ["" ("Substring") "error: DLL connect interface function failed. " ("Substring")] -> w880
                tunnel: w869 -> [w894 _]
                tunnel: [w894 100 ("DLL I32 Return value")] -> w868
                frame False {
                }
                frame True {
                }
              }
              n313 = Number To Decimal String(number=w868) -> (decimal integer string=w878:string)  [unwired: 1 out]
              n314 = Concatenate Strings("Open interface ", w886, w883, w880, w875, " Errorcode: " ("string"), w878) -> (w877:string)
            }
            frame True {
              n315 = Concatenate Strings("Open interface ", "error: Cannot load GCS DLL." ("Substring")) -> (w904:string)
            }
          }
          n316 = Bundle By Name(cluster=w860, "status"=TRUE, "code"=w862, "source"=w861) -> (w864:errorcluster)
        }
      }
      n317 = Unbundle By Name(w27) -> ("status"=w43:bool)
      n318 = case shown="False" w43 {
        tunnel: w9 -> [w828 _]
        tunnel: w27 -> [w831 w858]
        tunnel: [w830 w858] -> w7
        tunnel: [w829 ""] -> w29
        frame False {
          # "Clear interface"
          n319 = stacked-sequence {
            seq-local: [w834 _ _ _ _ _] -> [_ _ w840 _ _ _]
            seq-local: [_ _ w839 _ _ _] -> [_ _ _ w846 _ _]
            seq-local: [_ _ _ w845 _ _] -> [_ _ _ _ w849 _]
            seq-local: [_ _ _ _ w848 _] -> [_ _ _ _ _ w855]
            tunnel: w828 -> [w836 _ w842 w847 w852 w856]
            tunnel: [_ _ _ _ _ w854] -> w830
            tunnel: w831 -> [w833 _ _ _ _ _]
            tunnel: [_ _ _ w844 _ _] -> w829
            frame #0 {
              # "Clear Inter-\nface (no\ncommand)"
              n320 = call "PI Send String.vi"("System no."=w836, "String to send"="Interface clear", "Attach termination char.?"=FALSE ("Attach Linefeed?"), "error in"=w833) -> ("error out"=w834:errorcluster)  [unwired: 15 out]
            }
            frame #1 {
              n321 = Wait (ms)(milliseconds to wait=u32 10) -> ()  [unwired: 1 out]
            }
            frame #2 {
              n322 = call "PI Send String.vi"("System no."=w842, "String to send"="String to Send", "Attach termination char.?"=TRUE ("Attach Linefeed?"), "error in"=w840) -> ("error out"=w839:errorcluster)  [unwired: 15 out]
            }
            frame #3 {
              n323 = call "PI Receive String.vi"("System no."=w847, "Strip spaces?"=FALSE, "error in"=w846) -> ("String read"=w844:string, "error out"=w845:errorcluster)  [unwired: 15 out]
            }
            frame #4 {
              # "Clear error\nstatus"
              n324 = call "PI Send String.vi"("System no."=w852, "String to send"="err?" ("String to Send"), "Attach termination char.?"=TRUE ("Attach Linefeed?"), "error in"=w849) -> ("error out"=w848:errorcluster)  [unwired: 15 out]
            }
            frame #5 {
              n325 = call "PI Receive String.vi"("System no."=w856, "Strip spaces?"=FALSE, "error in"=w855) -> ("error out"=w854:errorcluster)  [unwired: 16 out]
            }
          }
        }
        frame True {
          # "Error!"
        }
      }
      n326 = case shown="No Error" w7 {
        selector: w7 -> [w44 w53]
        tunnel: [w49 w53] -> w8
        tunnel: w9 -> [w50 _]
        frame No Error {
          # "Create Semaphore reference\nand write in Global1"
          n327 = Number To Decimal String(number=w50) -> (decimal integer string=w51:string)  [unwired: 1 out]
          n328 = global read "Global1.vi" "PI Semaphore"() -> (w47:string[])
          n329 = Concatenate Strings("PI_GCSLabVIEW_Semaphore_", w51) -> (w45:string)
          n330 = Decrement(x=w50) -> (x-1=w46:i32)
          n331 = call <vilib>:"Obtain Semaphore Reference.vi"("error in (no error)"=w44, "name (unnamed)"=w45) -> ("error out"=w49:errorcluster)  [unwired: 1 in, 4 out]
          n332 = Replace Array Subset(array=w47, new element=w45, index=w46) -> (w48:string[])
          n333 = global write "Global1.vi" "PI Semaphore"(w48) -> ()
        }
        frame Error {
        }
      }
    }
    frame Error {
      (unwired) 0 ("error code")
    }
  }
  "error out" <- w4
  "String read" <- w5
